vi "Test DAQ OPC and Robot.vi"(7 "error in":errorcluster) -> (0 "error out":errorcluster)   [LabVIEW 2013]
uses:
  SLL DAQ Engine/Software/Source Code/Sub VIs/DAQ Engine/Controls/SLL DE List of Digital Inputs.ctl
  SLL DAQ Engine/Software/Source Code/Sub VIs/DAQ Engine/Controls/SLL DE List of Digital Outputs.ctl
  Controls/ALTS-2015 Auto Program States.ctl
  Controls/ALTS-2015 Station Cluster.ctl
  Controls/ALTS-2015 Serial DB Details.ctl
  Controls/ALTS-2015 Serial Details.ctl
  Controls/ALTS-2015 Robot Tasks.ctl
  Controls/ALTS-2015 Robot FIFO Queue Options.ctl
  Controls/ALTS-2015 Task at Station Options.ctl
  Controls/ALTS-2015 LV2GBL Station Info Options.ctl
  SLL DAQ Engine/Software/Source Code/Sub VIs/DAQ Engine/Controls/SLL DE DI Global Options.ctl
  SLL DAQ Engine/Software/Source Code/Sub VIs/DAQ Engine/Controls/SLL DE DO Global Options.ctl
  Sub VIs/OPC Engine/Controls/ALTS-2015 OPC Write Global Options.ctl
  Sub VIs/OPC Engine/Controls/ALTS-2015 OPC Write Registers.ctl
  Sub VIs/OPC Engine/Controls/ALTS-2015 OPC Read Registers.ctl
  Sub VIs/OPC Engine/Controls/ALTS-2015 OPC Read Global Options.ctl
  Sub VIs/Robot Controller Queue/ALTS-2015 Robot Cotroller Options.ctl
  Globals/ALTS-2015 Global Variables.vi
panel:
  in  "Tab Control":T1(tab)
  out "History":string
  in  "STATION1 Start":bool
  in  "STATION1 Stop":bool
  in  "STATION1 Clamped":bool
  in  "STATION1 Test Type":T2(ring)=enum."Test Type 4"
  in  "STATION1 TC PASS":bool
  in  "STATION1 TC FAIL":bool
  in  "STATION1 Start DO":bool
  in  "Start Test":bool
  in  "Stop Test":bool
  in  "Scan Trigger":bool
  in  "Station No Start Stop Test":T3(ring)
  in  "Robot Available":bool
  out "Task Available for Robot?":bool
  out "New Serial Task?":bool
  out "Serial Adapter Plate Size":dbl
  out "Serial Displacement Size":dbl
  out "Serial Flange Size":dbl
  out "Test Result":bool
  out "Station Number":T3(ring)
  out "Rerun?":bool
  out "Invalid Serial Number":bool
  in  "PC ACK":bool
  in  "STATION3 Start":bool
  in  "STATION3 Stop":bool
  in  "STATION3 Clamped":bool
  in  "STATION3 Test Type":T2(ring)=enum."Test Type 4"
  in  "STATION3 TC PASS":bool
  in  "STATION3 TC FAIL":bool
  in  "STATION3 Start DO":bool
  in  "STATION2 Start":bool
  in  "STATION2 Stop":bool
  in  "STATION2 Clamped":bool
  in  "STATION2 Test Type":T2(ring)=enum."Test Type 4"
  in  "STATION2 TC PASS":bool
  in  "STATION2 TC FAIL":bool
  in  "STATION2 Start DO":bool
  in  "STATION4 Start":bool
  in  "STATION4 Stop":bool
  in  "STATION4 Clamped":bool
  in  "STATION4 Test Type":T2(ring)=enum."Test Type 4"
  in  "STATION4 TC PASS":bool
  in  "STATION4 TC FAIL":bool
  in  "STATION4 Start DO":bool
  in  "STATION1 Select Test":bool
  in  "STATION2 Select Test":bool
  in  "STATION3 Select Test":bool
  in  "STATION4 Select Test":bool
  out "Station No.":string[](array[string])=["Station 1", "Station 2", "Station 3", "Station 4"]
  out "Test Type":i32[](array[numeric])
  in  "STATION2 Stop DO":bool
  in  "STATION1 Stop DO":bool
  in  "STATION3 Stop DO":bool
  in  "STATION4 Stop DO":bool
  in  "STATION1 Light Indicator":enum16{"IDLE", "Test Running", "Pass", "Fail"}(ring)
  in  "STATION2 Light Indicator":enum16{"IDLE", "Test Running", "Pass", "Fail"}(ring)
  in  "STATION3 Light Indicator":enum16{"IDLE", "Test Running", "Pass", "Fail"}(ring)
  in  "STATION4 Light Indicator":enum16{"IDLE", "Test Running", "Pass", "Fail"}(ring)
  in  "Clear History":bool
  out "Serial Height":dbl
  out "Load Decision":dbl
  out "Cart Insert":dbl
  in  "Flush FIFO Queue":bool
  in  "Trigger Robot Controller State":bool
  in  "Roboto Controller State to Execute":T4=enum."Write Task Available for Robot"
  out "Load Serial Tasks":T5[](array[typedef])
  out "Invalid Serial Tasks":T5[](array[typedef])
  out "Rerun Serial Tasks":T5[](array[typedef])
  out "Unload Serial Tasks":T5[](array[typedef])
  out "# Unload Serial Tasks":i32
  out "# Rerun Serial Tasks":i32
  out "# Invalid Serial Tasks":i32
  out "# Load Serial Tasks":i32
  in  "New Serial Task Data":T9
  in  "Rerun Task Data":T10
  in  "Enqueue Invalid Serial":bool
  in  "Unload Task Data":T11
  out "All FIFO Elements":T5[](array[typedef])
  out "Current Station 1 Task":T5
  out "Current Station 2 Task":T5
  out "Current Station 3 Task":T5
  out "Current Station 4 Task":T5
  in  "Cart_Insert DS":dbl
  in  "Load_Decision DS":dbl
  in  "Serial_Height DS":dbl format="%.2g"
  in  "PC_ACK_Read_Tags DS":dbl
  out "DO Channel Name":T12
  in  "Invalid_SNo DS":dbl
  in  "Station_No_Start_Stop_Test DS":dbl
  in  "Start_Test DS":dbl
  in  "Rerun DS":dbl
  in  "Station_Number DS":dbl
  in  "Test_Result DS":dbl
  in  "Serial_Flange_Size DS":dbl
  in  "Serial_Displacement_Size DS":dbl
  in  "Serial_Adapter_Size DS":dbl
  in  "New_Serial DS":dbl
  in  "Scan_Trigger DS":dbl
  in  "Stop_Test DS":dbl
  in  "Task_Available_for_Robot DS":dbl
  in  "Robot_Available DS":dbl
  in  "DI Array":bool[](array[boolean])=[FALSE, FALSE, FALSE, FALSE, FALSE, FALSE, FALSE, FALSE, FALSE, FALSE, FALSE, FALSE, FALSE, FALSE, FALSE, FALSE, FALSE, FALSE, FALSE, FALSE, FALSE, FALSE, FALSE, FALSE, FALSE, FALSE, FALSE, FALSE]
  in  "DI Channel Name Array":T13[](array[typedef])=[enum."STATION1_START", enum."STATION1_STOP", enum."STATION1_CLAMPED", enum."STATION1_TC_PASS", enum."STATION1_TC_FAIL", enum."STATION1_TTA", enum."STATION1_TTB", enum."STATION2_START", enum."STATION2_STOP", enum."STATION2_CLAMPED", enum."STATION2_TC_PASS", enum."STATION2_TC_FAIL", enum."STATION2_TTA", enum."STATION2_TTB", enum."STATION3_START", enum."STATION3_STOP", enum."STATION3_CLAMPED", enum."STATION3_TC_PASS", enum."STATION3_TC_FAIL", enum."STATION3_TTA", enum."STATION3_TTB", enum."STATION4_START", enum."STATION4_STOP", enum."STATION4_CLAMPED", enum."STATION4_TC_PASS", enum."STATION4_TC_FAIL", enum."STATION4_TTA", enum."STATION4_TTB"]
  out "DO Channel Name Array":T12[](array[typedef])=[enum."STATION1_START TEST", enum."STATION1_STOP TEST", enum."STATION1_LIGHT1", enum."STATION1_LIGHT2", enum."STATION1_LIGHT3", enum."STATION1_SELECT_TEST", enum."STATION2_START TEST", enum."STATION2_STOP TEST", enum."STATION2_LIGHT1", enum."STATION2_LIGHT2", enum."STATION2_LIGHT3", enum."STATION2_SELECT_TEST", enum."STATION3_START TEST", enum."STATION3_STOP TEST", enum."STATION3_LIGHT1", enum."STATION3_LIGHT2", enum."STATION3_LIGHT3", enum."STATION3_SELECT_TEST", enum."STATION4_START TEST", enum."STATION4_STOP TEST", enum."STATION4_LIGHT1", enum."STATION4_LIGHT2", enum."STATION4_LIGHT3", enum."STATION4_SELECT_TEST"]
  out "DO Array":bool[](array[boolean])=[FALSE, FALSE, FALSE, FALSE, TRUE, FALSE, FALSE, FALSE, FALSE, FALSE, TRUE, FALSE, FALSE, FALSE, FALSE, FALSE, FALSE, FALSE, FALSE, FALSE, FALSE, FALSE, FALSE, FALSE]
  in  "DI Channel Name":T13
  # "ALTS-2015 Auto Mode Troubleshooter"
  # "Simulation VI to send DI Status and reads the DO output"
  # "Write Tags\nPC Writes to PLC\nPLC can only read these tags"
  # "Read Tags\nPC Reads from PLC"
  # "Test Type1: TTA:1, TTB: 0;\nTest Type2: TTA:0, TTB: 1;\nTest Type3: TTA:1, TTB: 1;\nTest Type4: TTA:0, TTB: 0;"
  # "IDLE : \t\t100\nTest Running:\t 010\nPass\t\t110\nFail\t\t101"
  # "STATION  1"
  # "STATION  2"
  # "Write Tags\nPC Writes to PLC\nPLC can only read these tags"
  # "Read Tags\nPC Reads from PLC"
  # "DI"
  # "DO"
  # "DI"
  # "DO"
  # "STATION  3"
  # "STATION  4"
  # "DI"
  # "DO"
  # "DI"
  # "DO"
  # "Invalid Serial Task Data"
  # "This tab indicates the tasks being executed at different station"
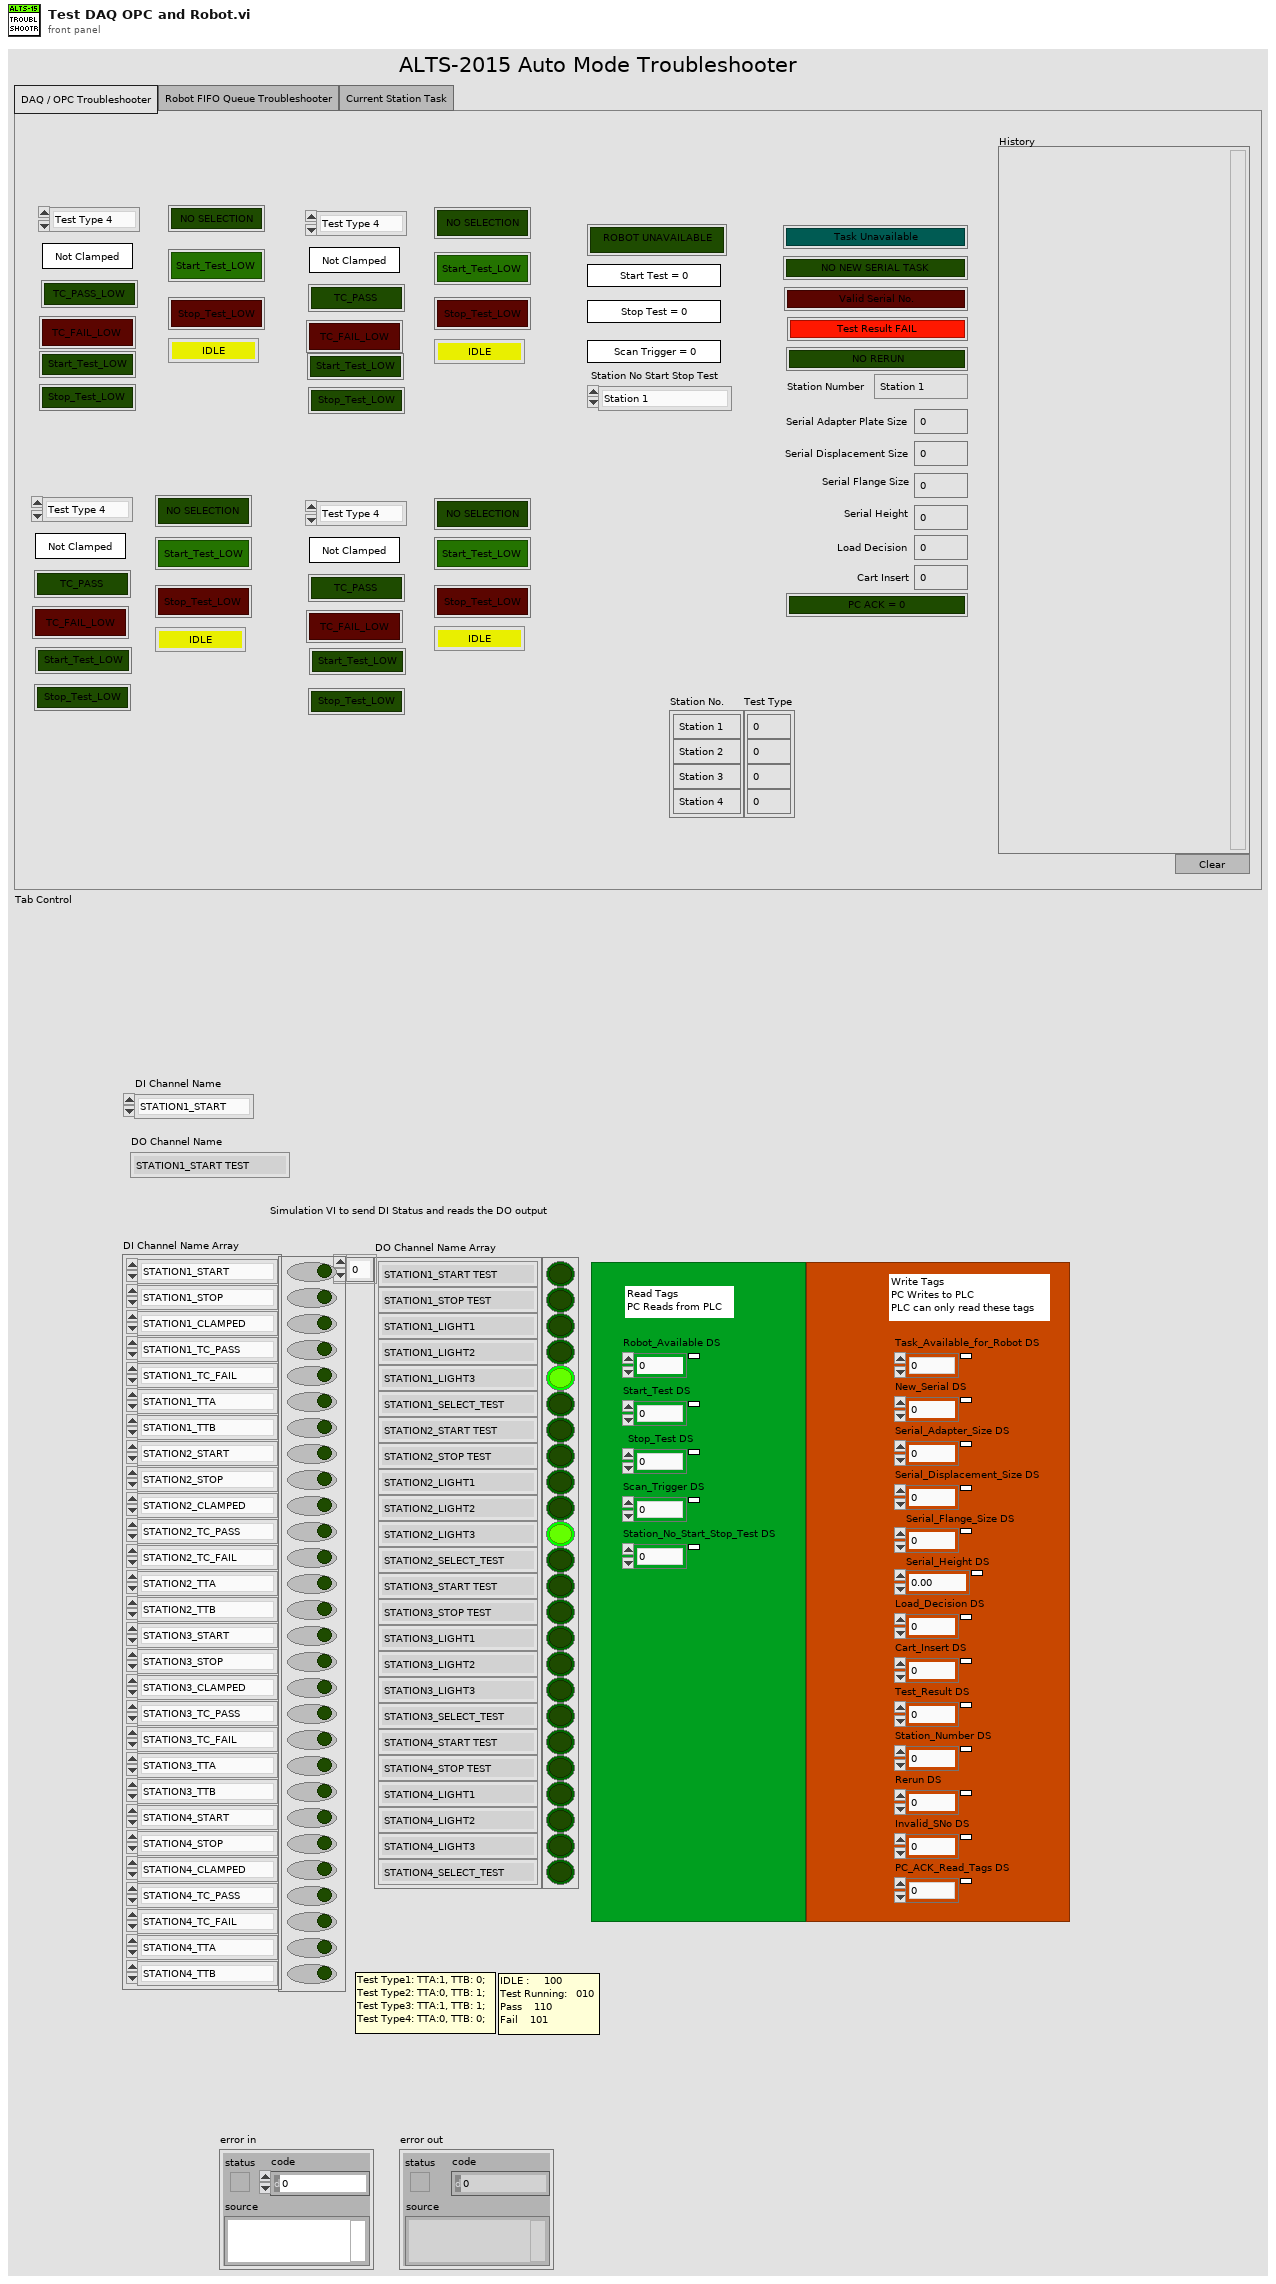
[diagram p1: front panel]
types:
  T1 = enum32{"DAQ / OPC Troubleshooter", "Robot FIFO Queue Troubleshooter", "Current Station Task"}
  T2 = enum16{"Test Type 1", "Test Type 2", "Test Type 3", "Test Type 4"}
  T3 = enum16{"Station 1", "Station 2", "Station 3", "Station 4"}
  T4 = typedef "ALTS-2015 Auto Program States.ctl" = enum16{"<------ Robot Handler States ------>", "Wait for Robot Availability", "Check Last Task by Robot", "Wait & Read Task from Queue", "Write New Task Details to Robot", "Write Task Available for Robot", "Check Robot for Unavailbilty", "Write Task Unavailable for Robot", "<------------ Other ------------>", "Error", "Exit"}
  T5 = typedef "ALTS-2015 Serial Details.ctl" = cluster{"Robot Task":T6, "Serial No":string, "New Serial?":bool, "Station # Unload":T7, "Last Test Result":bool, "Rerun?":bool, "Station # Rerun":T7, "Invalid Serial?":bool, "Serial Details":T8}
  T6 = typedef "ALTS-2015 Robot Tasks.ctl" = enum16{"Load", "Unload", "Rerun", "Invalid Serial"}
  T7 = typedef "ALTS-2015 Station Cluster.ctl" = enum16{"Station 1", "Station 2", "Station 3", "Station 4"}
  T8 = typedef "ALTS-2015 Serial DB Details.ctl" = cluster{"Adapter Plate Size":i32, "Air Leak Test Type ":i32, "Displacement Size":i32, "Flange Size":i32, "Height":i32, "Load Decision":i32, "Cart Insert":i32}
  T9 = cluster{"New Serial Details":T8, "Enqueue New Serial Task":bool}
  T10 = cluster{"Station # Rerun":T7, "Enqueue Rerun Task":bool}
  T11 = cluster{"Last Test Result":bool, "Station # Unload":T7, "Load Decision":i32, "Enqueue Unload Task":bool}
  T12 = typedef "SLL DE List of Digital Outputs.ctl" = enum16{"STATION1_START TEST", "STATION1_STOP TEST", "STATION1_LIGHT1", "STATION1_LIGHT2", "STATION1_LIGHT3", "STATION1_SELECT_TEST", "STATION2_START TEST", "STATION2_STOP TEST", "STATION2_LIGHT1", "STATION2_LIGHT2", "STATION2_LIGHT3", "STATION2_SELECT_TEST", "STATION3_START TEST", "STATION3_STOP TEST", "STATION3_LIGHT1", "STATION3_LIGHT2", "STATION3_LIGHT3", "STATION3_SELECT_TEST", "STATION4_START TEST", "STATION4_STOP TEST", "STATION4_LIGHT1", "STATION4_LIGHT2", "STATION4_LIGHT3", "STATION4_SELECT_TEST"}
  T13 = typedef "SLL DE List of Digital Inputs.ctl" = enum16{"STATION1_START", "STATION1_STOP", "STATION1_CLAMPED", "STATION1_TC_PASS", "STATION1_TC_FAIL", "STATION1_TTA", "STATION1_TTB", "STATION2_START", "STATION2_STOP", "STATION2_CLAMPED", "STATION2_TC_PASS", "STATION2_TC_FAIL", "STATION2_TTA", "STATION2_TTB", "STATION3_START", "STATION3_STOP", "STATION3_CLAMPED", "STATION3_TC_PASS", "STATION3_TC_FAIL", "STATION3_TTA", "STATION3_TTB", "STATION4_START", "STATION4_STOP", "STATION4_CLAMPED", "STATION4_TC_PASS", "STATION4_TC_FAIL", "STATION4_TTA", "STATION4_TTB"}
  T14 = enum32{"No PSP", "Read", "Write", "Write & Read"}
  T15 = typedef "ALTS-2015 INI Configuration Cluster.ctl" = cluster{"Application":cluster{"Rerun Count":i32, "Workorder No":string}, "Station Details":cluster{"Sensor Name 1":string, "Sensor Name 2":string, "Sensor Name 3":string, "Sensor Name 4":string, "Station1 Enable":bool, "Station2 Enable":bool, "Station3 Enable":bool, "Station4 Enable":bool}, "Database":cluster{"Database Connection Link":path, "Result Procedure":string, "User":string, "Password":string, "Prompt":bool, "Station 1 LT Result DB DSN Path":path, "Station 2 LT Result DB DSN Path":path, "Station 3 LT Result DB DSN Path":path, "Station 4 LT Result DB DSN Path":path, "AirLeakTestResult Procedure":string, "Serial Details Procedure":string}, "Simulation":cluster{"Simulate DAQ Hardware":bool, "Simulate Result DB Write":bool, "Simulate Scanner":bool, "Simulate OPC":bool, "Simulate Serial Details DB":bool, "Simulate Result DB":bool, "Simulate Scanner DB Path":path, "Simulate Serial Details DB Path":path, "Simulate Result DB Path":path}, "Barcode Scanner1":cluster{"Scanner IP":string, "Scanner Port":u16, "#Bytes to Read":i32}, "Barcode Scanner2":cluster{"Enabled?":bool, "Scanner IP":string, "Scanner Port":u16, "#Bytes to Read":i32}}
  T16 = typedef "SLL DE DO Global Options.ctl" = enum16{"Init", "Write Line", "Write Array", "Write Full Status", "Read Line", "Read Array", "Read Full Status", "Restart DO", "Send to Safe Mode", "Stop DO"}
  T17 = typedef "SLL DE DI Global Options.ctl" = enum16{"Init", "Write Line", "Write Array", "Read Line", "Read Array", "Read Full Status", "Write Full Status"}
  T18 = typedef "ALTS-2015 LV2GBL Station Info Options.ctl" = enum16{"Init", "Read", "Read All", "Write Sensor ID", "Write  Work Order", "Write Serial Number", "Write Test Data", "Write Station Status", "Write Station Occupancy", "Write Station Test Type", "Write Rerun", "Write Load Decision", "Write Robot Action", "Clear All", "Clear Test Result"}
  T19 = typedef "ALTS-2015 OPC Read Global Options.ctl" = enum16{"Init", "Write Value", "Write Array", "Read Value", "Read Array", "Read All"}
  T20 = typedef "ALTS-2015 OPC Write Global Options.ctl" = enum16{"Init", "Write Value", "Write Array", "Read Value", "Read Array", "Read All"}
  T21 = typedef "ALTS-2015 Robot Cotroller Options.ctl" = enum16{"Init", "Enqueue State", "Enqueue State in Opposite End", "Dequeue State", "Exit"}
  T22 = typedef "ALTS-2015 Robot FIFO Queue Options.ctl" = enum16{"Init", "Enqueue", "Dequeue", "Get Queue Elements", "Flush", "Destroy"}
  T23 = typedef "ALTS-2015 OPC Read Registers.ctl" = enum16{"Robot_Available", "Start_Test", "Stop_Test", "Scan_Trigger", "Station_No_Start_Stop_Test"}
  T24 = typedef "ALTS-2015 OPC Write Registers.ctl" = enum16{"Task_Available_for_Robot", "New_Serial", "Serial_Adapter_Size", "Serial_Displacement_Size", "Serial_Flange_Size", "Serial_Height", "Serial_LoadDecision", "Serial_CartInsert", "Test_Result", "Station_Number", "Rerun", "Invalid_SNo", "PC_ACK_Read_Tags"}
  T25 = typedef "ALTS-2015 Station Details.ctl" = cluster{"Station Number":string, "Work Order Number":string, "Sensor Name":string, "Pressure (PSI)":string, "Flow (SCCM)":string, "Test Time ":string, "Test Result":string, "Serial Number":string, "Station Status":T26, "SW assigned UUT":bool, "Rerun Count":i32, "Test Type":i32, "Load Decision":i32, "Robot Action":T27}
  T26 = typedef "ALTS-2015 Status Ring Indicator.ctl" = u16
  T27 = typedef "ALTS-2015 Robot Actions.ctl" = enum16{"Loading...", "Unloading...", "Reruning...", "No Action"}
  T28 = typedef "ALTS-2015 Task at Station Options.ctl" = enum16{"Init", "Write", "Read All", "Read"}
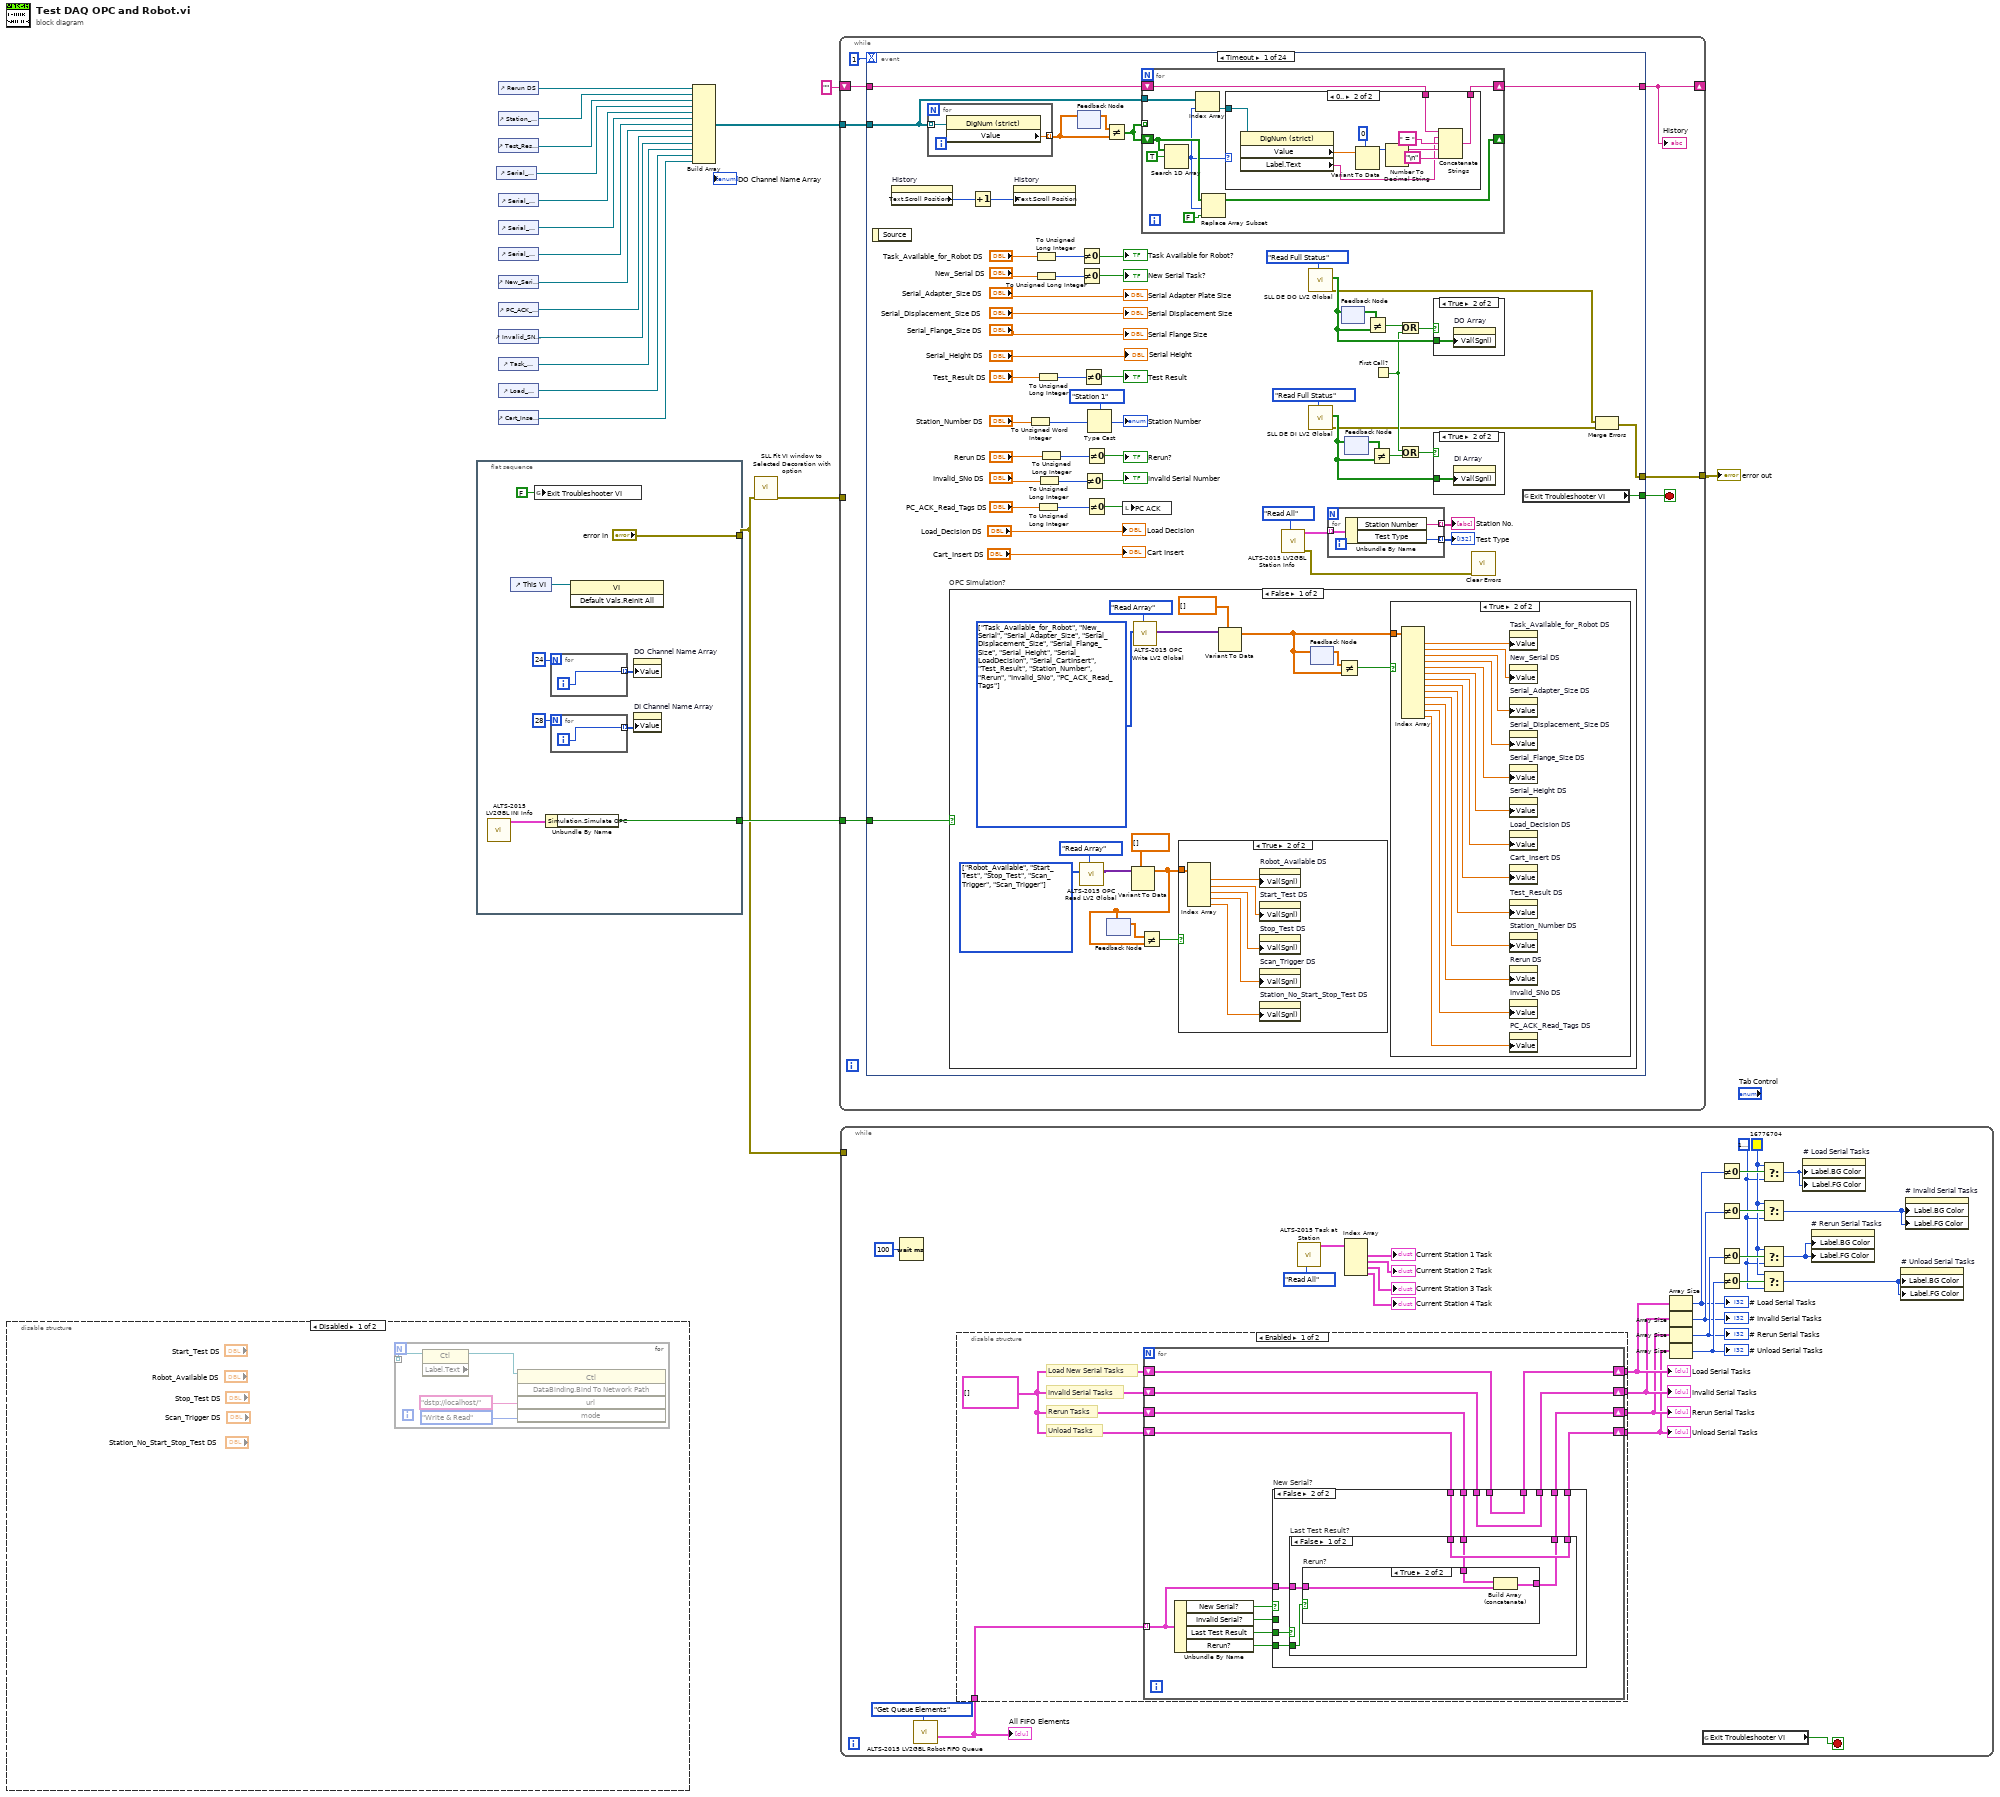
[diagram p0: block diagram]
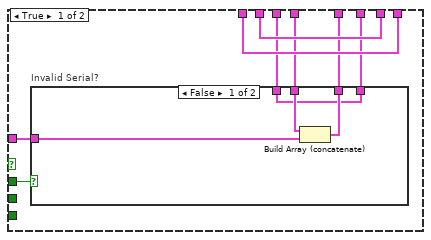
[diagram p2: hidden frame]
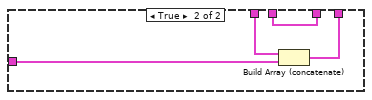
[diagram p3: hidden frame]
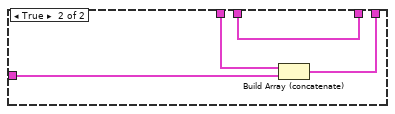
[diagram p5: hidden frame]
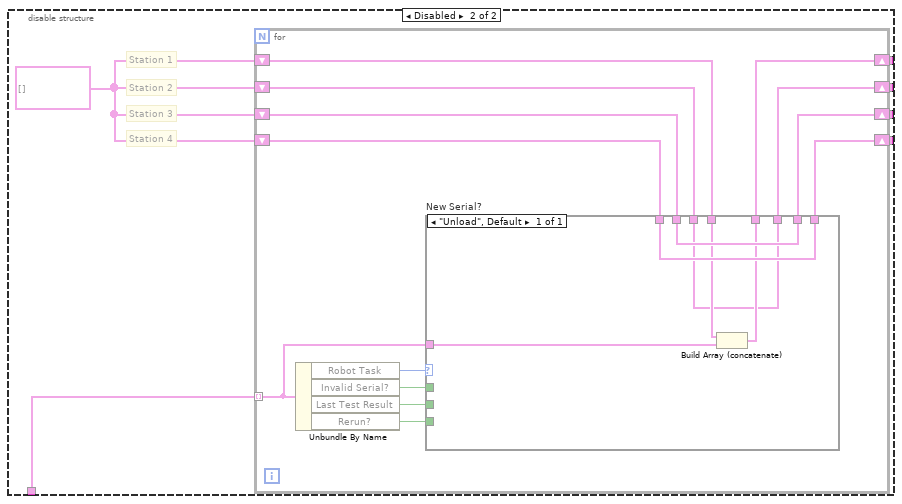
[diagram p6: hidden frame]
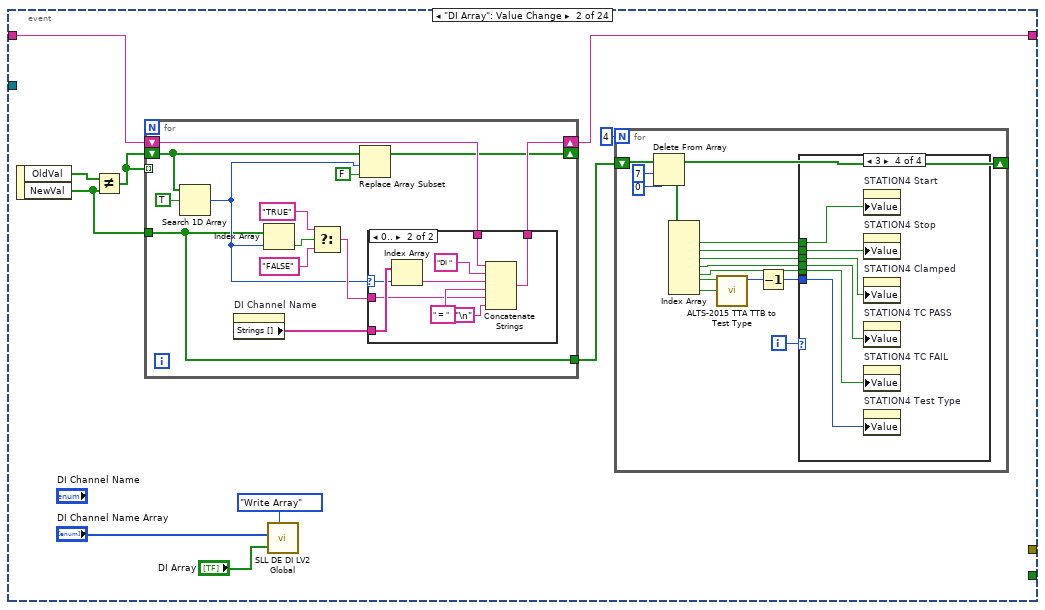
[diagram p13: hidden frame]
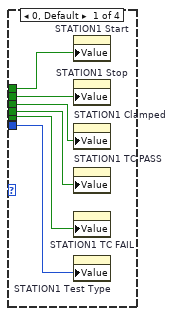
[diagram p14: hidden frame]
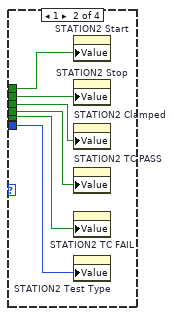
[diagram p15: hidden frame]
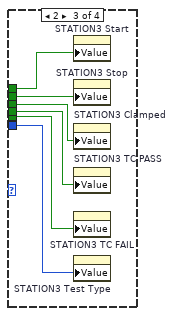
[diagram p16: hidden frame]
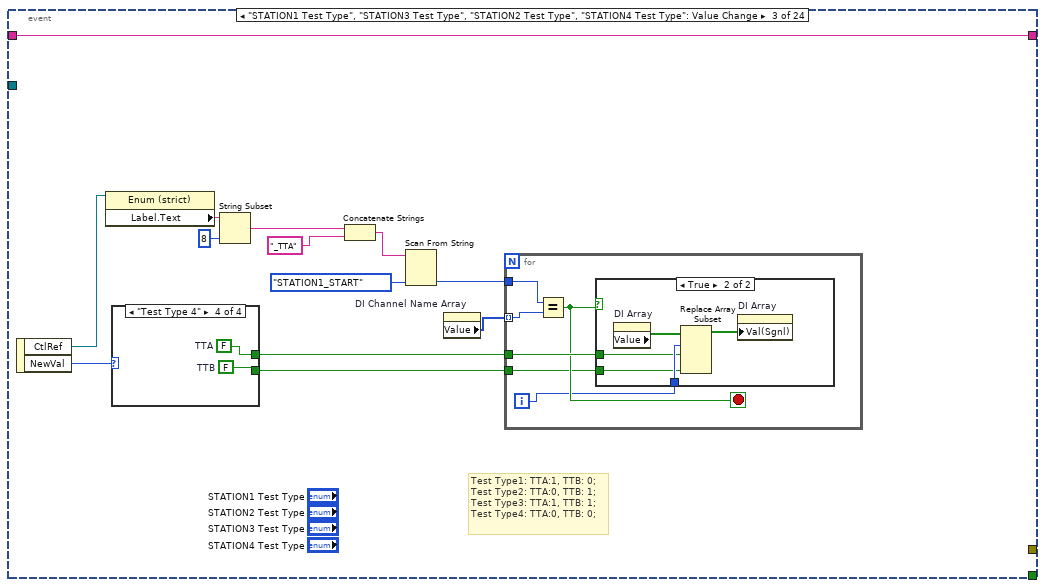
[diagram p18: hidden frame]
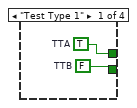
[diagram p19: hidden frame]
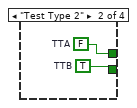
[diagram p20: hidden frame]
diagram:
  n1 = disable-structure shown="Disabled" {
    frame Disabled {
      n2 = for {
        tunnel: [w24] -> w20 mode=indexing
        n3 = property class="Ctl" props=["Label", "Text"](reference=w24) -> (reference out=w21:refnum<vi>)  [unwired: 1 in, 2 out]
        n4 = invoke on="Invoke Node" class="Ctl" method="DataBinding.Bind To Network Path"(reference=w21, "url"="dstp://localhost/" ("URL"), "mode"=T14."Write & Read" ("Mode")) -> ()  [unwired: 2 in, 5 out]
      }
    }
    frame Enabled {
    }
  }
  n5 = flat-sequence {
    tunnel: ["error in"] -> w1
    tunnel: [w25] -> w2
    frame #0 {
      n6 = call "ALTS-2015 LV2GBL INI Info.vi"() -> ("Configuration Cluster Out"=w26:T15)  [unwired: 10 in, 1 out]
      n7 = control-ref of="This VI"() -> (w31:refnum<vi>)
      n8 = global write "ALTS-2015 Global Variables.vi" "Exit Troubleshooter VI"(FALSE ("Exit Troubleshooter VI")) -> ()
      n9 = Unbundle By Name(w26) -> ("Simulation.Simulate OPC"=w25:bool)
      n10 = for {
        N: 24 -> [_]
        tunnel: [w35] -> w27 mode=indexing
        i -> [w35]
      }
      n11 = for {
        N: 28 -> [_]
        tunnel: [w34] -> w30 mode=indexing
        i -> [w34]
      }
      n12 = invoke class="VI" method="Default Vals.Reinit All"(reference=w31) -> ()  [unwired: 2 in, 3 out]
      n13 = property on="DO Channel Name Array" class="Arr (strict)"("Value"=w27) -> ()  [unwired: 2 in, 2 out]
      n14 = property on="DI Channel Name Array" class="Arr (strict)"("Value"=w30) -> ()  [unwired: 2 in, 2 out]
    }
  }
  n15 = control-ref of="Serial_Flange_Size DS"() -> (w17:refnum<vi>)
  n16 = control-ref of="Rerun DS"() -> (w14:refnum<vi>)
  n17 = control-ref of="Station_Number DS"() -> (w15:refnum<vi>)
  n18 = control-ref of="Test_Result DS"() -> (w16:refnum<vi>)
  n19 = control-ref of="Serial_Displacement_Size DS"() -> (w18:refnum<vi>)
  n20 = control-ref of="Serial_Adapter_Size DS"() -> (w19:refnum<vi>)
  n21 = control-ref of="Serial_Height DS"() -> (w9:refnum<vi>)
  n22 = control-ref of="New_Serial DS"() -> (w8:refnum<vi>)
  n23 = control-ref of="PC_ACK_Read_Tags DS"() -> (w7:refnum<vi>)
  n24 = control-ref of="Invalid_SNo DS"() -> (w6:refnum<vi>)
  n25 = control-ref of="Task_Available_for_Robot DS"() -> (w5:refnum<vi>)
  n26 = control-ref of="Load_Decision DS"() -> (w4:refnum<vi>)
  n27 = control-ref of="Cart_Insert DS"() -> (w3:refnum<vi>)
  n28 = Build Array(w14, w15, w16, w17, w18, w19, w9, w8, w7, w6, w5, w4, w3) -> (w11:refnum<vi>[])
  n29 = call "SLL Fit VI window to Selected Decoration with option.vi"("error in (no error)"=w1) -> ("error out"=w13:errorcluster)  [unwired: 9 in, 1 out]
  n30 = while {
    tunnel: w13 -> [_]
    tunnel: [w40] -> w10
    shift-right: [w38] -> _
    shift-left: "" -> [w39]
    tunnel: w11 -> [w37]
    tunnel: w2 -> [w36]
    stop <- w42 stop-if-true
    n31 = event shown="[0] Timeout" {
      selector: _ -> [_ _ _ _ _ _ _ _ _ _ _ _ _ _ _ _ _ _ _ _ _ _ _ _]
      dyn-events: _ -> [_ _ _ _ _ _ _ _ _ _ _ _ _ _ _ _ _ _ _ _ _ _ _ _]
      timeout: 1 -> [_ _ _ _ _ _ _ _ _ _ _ _ _ _ _ _ _ _ _ _ _ _ _ _]
      tunnel: [w77 _ _ _ _ _ _ _ _ _ _ _ _ _ _ _ _ _ _ _ _ _ _ _] -> w42
      tunnel: [w44 _ _ _ _ _ _ _ _ _ _ _ _ _ _ _ _ _ _ _ _ _ _ _] -> w40
      tunnel: [w65 w161 w233 w265 w285 w305 w325 w345 w366 w476 w511 w518 w521 w524 w527 w530 w534 w535 w538 w545 w553 w562 w570 ""] -> w38
      tunnel: w39 -> [w64 w162 w233 w265 w285 w305 w325 w345 w367 w476 w512 w518 w521 w524 w527 w530 w534 w535 w538 w545 w553 w562 w570 _]
      tunnel: w37 -> [w63 _ _ _ _ _ _ _ _ _ _ _ _ _ _ _ _ _ _ _ _ _ _ _]
      tunnel: w36 -> [w49 _ _ _ _ _ _ _ _ _ _ _ _ _ _ _ _ _ _ _ _ _ _ _]
      event Timeout {
        n32 = event-data() -> ()  [unwired: 1 in, 1 out]
        n33 = property on="History" class="Str"() -> ("Text.Scroll Position"=w62:u32)  [unwired: 2 in, 2 out]
        n34 = for {
          tunnel: w63 -> [w156] mode=indexing
          tunnel: [w155] -> w53 mode=indexing
          n35 = property class="DigNum (strict)"(reference=w156) -> ("Value"=w155:dbl)  [unwired: 1 in, 2 out]
        }
        n36 = case "OPC Simulation?" shown="False" w49 {
          frame False {
            w109 = T23[] [enum."Robot_Available", enum."Start_Test", enum."Stop_Test", enum."Scan_Trigger", enum."Scan_Trigger"] items=["Robot_Available", "Start_Test", "Stop_Test", "Scan_Trigger", "Station_No_Start_Stop_Test"] ("OPC Read Register Array")
            w110 = T24[] [enum."Task_Available_for_Robot", enum."New_Serial", enum."Serial_Adapter_Size", enum."Serial_Displacement_Size", enum."Serial_Flange_Size", enum."Serial_Height", enum."Serial_LoadDecision", enum."Serial_CartInsert", enum."Test_Result", enum."Station_Number", enum."Rerun", enum."Invalid_SNo", enum."PC_ACK_Read_Tags"] items=["Task_Available_for_Robot", "New_Serial", "Serial_Adapter_Size", "Serial_Displacement_Size", "Serial_Flange_Size", "Serial_Height", "Serial_LoadDecision", "Serial_CartInsert", "Test_Result", "Station_Number", "Rerun", "Invalid_SNo", "PC_ACK_Read_Tags"] ("OPC Write Register Array")
            n37 = call "ALTS-2015 OPC Read LV2 Global.vi"("Options"=ALTS-2015_OPC_Read_Global_Options."Read Array", "OPC Read Register Array"=w109) -> ("OPC Read Register Array Value"=w106:variant[])  [unwired: 7 in, 2 out]
            n38 = feedback #1() -> (w105:dbl[])  [unwired: 1 in]
            n39 = Variant To Data(type=dbl[] [], Variant=w106) -> (data=w103:dbl[])  [unwired: 1 in, 1 out]
            n40 = feedback-in #1(w103) -> ()
            n41 = call "ALTS-2015 OPC Write LV2 Global.vi"("Options"=ALTS-2015_OPC_Write_Global_Options."Read Array", "OPC Write Register Array"=w110) -> ("OPC Read Register Array Value"=w112:variant[])  [unwired: 7 in, 2 out]
            n42 = Not Equal?(x=w105, y=w103) -> (x != y?=w101:bool)
            n43 = case shown="True" w101 {
              tunnel: w103 -> [_ w128]
              frame False {
              }
              frame True {
                n44 = Index Array(array=w128) -> (element #1=w133:dbl, element #2=w132:dbl, element #3=w131:dbl, element #4=w130:dbl, element #5=w129:dbl)  [unwired: 5 in]
                n45 = property on="Robot_Available DS" class="DigNum (strict)"("Val(Sgnl)"=w133) -> ()  [unwired: 2 in, 2 out]
                n46 = property on="Start_Test DS" class="DigNum (strict)"("Val(Sgnl)"=w132) -> ()  [unwired: 2 in, 2 out]
                n47 = property on="Stop_Test DS" class="DigNum (strict)"("Val(Sgnl)"=w131) -> ()  [unwired: 2 in, 2 out]
                n48 = property on="Scan_Trigger DS" class="DigNum (strict)"("Val(Sgnl)"=w130) -> ()  [unwired: 2 in, 2 out]
                n49 = property on="Station_No_Start_Stop_Test DS" class="DigNum (strict)"("Val(Sgnl)"=w129) -> ()  [unwired: 2 in, 2 out]
              }
            }
            n50 = Variant To Data(type=dbl[] [], Variant=w112) -> (data=w102:dbl[])  [unwired: 1 in, 1 out]
            n51 = feedback #2() -> (w104:dbl[])  [unwired: 1 in]
            n52 = feedback-in #2(w102) -> ()
            n53 = Not Equal?(x=w104, y=w102) -> (x != y?=w100:bool)
            n54 = case shown="True" w100 {
              tunnel: w102 -> [_ w114]
              frame False {
              }
              frame True {
                n55 = Index Array(array=w114) -> (element #1=w115:dbl, element #2=w116:dbl, element #3=w117:dbl, element #4=w118:dbl, element #5=w119:dbl, element #6=w120:dbl, element #7=w121:dbl, element #8=w122:dbl, element #9=w123:dbl, element #10=w124:dbl, element #11=w125:dbl, element #12=w126:dbl, element #13=w127:dbl)  [unwired: 13 in]
                n56 = property on="Task_Available_for_Robot DS" class="DigNum (strict)"("Value"=w115) -> ()  [unwired: 2 in, 2 out]
                n57 = property on="New_Serial DS" class="DigNum (strict)"("Value"=w116) -> ()  [unwired: 2 in, 2 out]
                n58 = property on="Serial_Adapter_Size DS" class="DigNum (strict)"("Value"=w117) -> ()  [unwired: 2 in, 2 out]
                n59 = property on="Serial_Displacement_Size DS" class="DigNum (strict)"("Value"=w118) -> ()  [unwired: 2 in, 2 out]
                n60 = property on="Serial_Flange_Size DS" class="DigNum (strict)"("Value"=w119) -> ()  [unwired: 2 in, 2 out]
                n61 = property on="Serial_Height DS" class="DigNum (strict)"("Value"=w120) -> ()  [unwired: 2 in, 2 out]
                n62 = property on="Load_Decision DS" class="DigNum (strict)"("Value"=w121) -> ()  [unwired: 2 in, 2 out]
                n63 = property on="Cart_Insert DS" class="DigNum (strict)"("Value"=w122) -> ()  [unwired: 2 in, 2 out]
                n64 = property on="Test_Result DS" class="DigNum (strict)"("Value"=w123) -> ()  [unwired: 2 in, 2 out]
                n65 = property on="Station_Number DS" class="DigNum (strict)"("Value"=w124) -> ()  [unwired: 2 in, 2 out]
                n66 = property on="Rerun DS" class="DigNum (strict)"("Value"=w125) -> ()  [unwired: 2 in, 2 out]
                n67 = property on="Invalid_SNo DS" class="DigNum (strict)"("Value"=w126) -> ()  [unwired: 2 in, 2 out]
                n68 = property on="PC_ACK_Read_Tags DS" class="DigNum (strict)"("Value"=w127) -> ()  [unwired: 2 in, 2 out]
              }
            }
          }
          frame True {
          }
        }
        n69 = Increment(x=w62) -> (x+1=w61:u32)
        n70 = property on="History" class="Str"("Text.Scroll Position"=w61) -> ()  [unwired: 2 in, 2 out]
        n71 = To Unsigned Word Integer(number="Station_Number DS") -> (unsigned 16bit integer=w80:u16)
        n72 = To Unsigned Long Integer(number="Task_Available_for_Robot DS") -> (unsigned 32bit integer=w97:u32)
        n73 = To Unsigned Long Integer(number="New_Serial DS") -> (unsigned 32bit integer=w96:u32)
        n74 = To Unsigned Long Integer(number="Test_Result DS") -> (unsigned 32bit integer=w90:u32)
        n75 = To Unsigned Long Integer(number="PC_ACK_Read_Tags DS") -> (unsigned 32bit integer=w58:u32)
        n76 = To Unsigned Long Integer(number="Invalid_SNo DS") -> (unsigned 32bit integer=w83:u32)
        n77 = To Unsigned Long Integer(number="Rerun DS") -> (unsigned 32bit integer=w86:u32)
        n78 = feedback-in #3(w53) -> ()
        n79 = feedback #3() -> (w52:dbl[])  [unwired: 1 in]
        n80 = Not Equal To 0?(x=w97) -> (x != 0?=→"Task Available for Robot?":bool)
        n81 = Not Equal To 0?(x=w96) -> (x != 0?=→"New Serial Task?":bool)
        n82 = Not Equal To 0?(x=w90) -> (x != 0?=→"Test Result":bool)
        n83 = Not Equal To 0?(x=w83) -> (x != 0?=→"Invalid Serial Number":bool)
        n84 = Not Equal To 0?(x=w86) -> (x != 0?=→"Rerun?":bool)
        n85 = Not Equal To 0?(x=w58) -> (x != 0?=w60:bool)
        n86 = Type Cast(type=T3."Station 1" ("Station Number"), x=w80) -> (*(type *) &x=→"Station Number":T3)
        n87 = Not Equal?(x=w52, y=w53) -> (x != y?=w66:bool[])
        n88 = local write "PC ACK"(w60) -> ()
        n89 = for {
          shift-right: [w138] -> _
          shift-left: w66 -> [w139]
          tunnel: w66 -> [_] mode=indexing
          shift-right: [w141] -> w65
          shift-left: w64 -> [w142]
          tunnel: w63 -> [w135]
          n90 = Search 1D Array(1D array=w139, element=TRUE) -> (index of element=w137:i32)  [unwired: 1 in]
          n91 = Index Array(array=w135, index=w137) -> (element=w140:refnum<vi>)
          n92 = Replace Array Subset(array=w139, new element=FALSE ("new element/subarray"), index=w137) -> (w138:bool[])
          n93 = case shown="0.." w137 {
            tunnel: [w144 w153] -> w141
            tunnel: w142 -> [w144 w152]
            tunnel: w140 -> [_ w147]
            frame -1, Default {
            }
            frame 0.. {
              n94 = property class="DigNum (strict)"(reference=w147) -> ("Value"=w151:dbl, "Label.Text"=w148:string)  [unwired: 1 in, 2 out]
              n95 = Variant To Data(type=0 ("concatenated string"), Variant=w151) -> (data=w145:i32)  [unwired: 1 in, 1 out]
              n96 = Number To Decimal String(number=w145) -> (decimal integer string=w150:string)  [unwired: 1 in]
              n97 = Concatenate Strings(w152, w148, " = " ("string"), w150, "\n") -> (w153:string)
            }
          }
        }
        n98 = call "ALTS-2015 LV2GBL Station Info.vi"("Options"=ALTS-2015_LV2GBL_Station_Info_Options."Read All") -> ("error out"=w72:errorcluster, "Station Info Array"=w74:T25[])  [unwired: 8 in, 1 out]
        n99 = call "SLL DE DO LV2 Global.vi"("DO Option"=SLL_DE_DO_Global_Options."Read Full Status") -> ("error out"=w43:errorcluster, "Digital Array Status"=w55:bool[])  [unwired: 7 in, 2 out]
        n100 = call "SLL DE DI LV2 Global.vi"("Option"=SLL_DE_DI_Global_Options."Read Full Status") -> ("error out"=w45:errorcluster, "Digital Array Status"=w70:bool[])  [unwired: 7 in, 2 out]
        n101 = for {
          tunnel: w74 -> [w160] mode=indexing
          tunnel: [w159] -> w76 mode=indexing
          tunnel: [w158] -> w75 mode=indexing
          n102 = Unbundle By Name(w160) -> ("Station Number"=w158:string, "Test Type"=w159:i32)
        }
        "Station No." <- w75
        "Test Type" <- w76
        n103 = feedback #4() -> (w56:bool[])  [unwired: 1 in]
        n104 = feedback-in #4(w55) -> ()
        n105 = feedback #5() -> (w68:bool[])  [unwired: 1 in]
        n106 = feedback-in #5(w70) -> ()
        n107 = Not Equal?(x=w56, y=w55) -> (x != y?=w57:bool)
        n108 = Not Equal?(x=w68, y=w70) -> (x != y?=w69:bool)
        n109 = First Call?() -> (First Call?: T/F=w46:bool)
        n110 = Or(x=w57, y=w46) -> (x .or. y?=w48:bool)
        n111 = Or(x=w46, y=w69) -> (x .or. y?=w47:bool)
        n112 = case shown="True" w48 {
          tunnel: w55 -> [_ w134]
          frame False {
          }
          frame True {
            n113 = property on="DO Array" class="Arr (strict)"("Val(Sgnl)"=w134) -> ()  [unwired: 2 in, 2 out]
          }
        }
        n114 = case shown="True" w47 {
          tunnel: w70 -> [_ w157]
          frame False {
          }
          frame True {
            n115 = property on="DI Array" class="Arr (strict)"("Val(Sgnl)"=w157) -> ()  [unwired: 2 in, 2 out]
          }
        }
        n116 = call <vilib>:"Clear Errors.vi"("error in (no error)"=w72) -> ()  [unwired: 6 in, 1 out]
        n117 = global read "ALTS-2015 Global Variables.vi" "Exit Troubleshooter VI"() -> (w77:bool)
        n118 = Merge Errors(w43, w45) -> (w44:errorcluster)
        "Serial Adapter Plate Size" <- "Serial_Adapter_Size DS"
        "Serial Displacement Size" <- "Serial_Displacement_Size DS"
        "Serial Flange Size" <- "Serial_Flange_Size DS"
        "Serial Height" <- "Serial_Height DS"
        "Cart Insert" <- "Cart_Insert DS"
        "Load Decision" <- "Load_Decision DS"
      }
      event "DI Array": Value Change {
        n119 = event-data() -> ("OldVal"=w164:bool[], "NewVal"=w163:bool[])  [unwired: 1 in]
        n120 = Not Equal?(x=w164, y=w163) -> (x != y?=w165:bool[])
        n121 = for {
          shift-right: [w215] -> _
          shift-left: w165 -> [w216]
          shift-right: [w221] -> w161
          shift-left: w162 -> [w220]
          tunnel: w165 -> [_] mode=indexing
          tunnel: w163 -> [w210]
          tunnel: [w210] -> w167
          n122 = Search 1D Array(1D array=w216, element=TRUE) -> (index of element=w212:i32)  [unwired: 1 in]
          n123 = property on="DI Channel Name" class="Enum (strict)"() -> ("Strings []"=w211:string[])  [unwired: 2 in, 2 out]
          n124 = Index Array(array=w210, index=w212) -> (element=w219:bool)
          n125 = Select(t="TRUE", s=w219, f="FALSE") -> (s? t:f=w213:string)
          n126 = Replace Array Subset(array=w216, new element=FALSE ("new element/subarray"), index=w212) -> (w215:bool[])
          n127 = case shown="0.." w212 {
            selector: w212 -> [_ w224]
            tunnel: w211 -> [_ w232]
            tunnel: [w223 w230] -> w221
            tunnel: w220 -> [w223 w229]
            tunnel: w213 -> [_ w227]
            frame -1, Default {
            }
            frame 0.. {
              n128 = Index Array(array=w232, index=w224) -> (element=w231:string)
              n129 = Concatenate Strings(w229, "DI " ("string"), w231, " = " ("string"), w227, "\n") -> (w230:string)
            }
          }
        }
        n130 = call "SLL DE DI LV2 Global.vi"("DI State Array"="DI Array", "Option"=SLL_DE_DI_Global_Options."Write Array", "DI Channel Name Array"="DI Channel Name Array") -> ()  [unwired: 5 in, 4 out]
        n131 = for {
          N: 4 -> [_]
          shift-right: [w181] -> _
          shift-left: w167 -> [w185]
          i -> [w172]
          n132 = Delete From Array(array=w185, length=7, index=0) -> (deleted portion=w182:bool[], array with subset deleted=w181:bool[])
          n133 = Index Array(array=w182) -> (element #1=w177:bool, element #2=w176:bool, element #3=w174:bool, element #4=w173:bool, element #5=w175:bool, element #6=w180:bool, element #7=w179:bool)  [unwired: 7 in]
          n134 = call "ALTS-2015 TTA TTB to Test Type.vi"("TTB"=w179, "TTA"=w180) -> ("Test Type"=w178:i32)  [unwired: 9 in]
          n135 = Decrement(x=w178) -> (x-1=w171:i32)
          n136 = case shown="3" w172 {
            tunnel: w171 -> [w191 w197 w203 w209]
            tunnel: w177 -> [w190 w196 w202 w208]
            tunnel: w176 -> [w189 w195 w201 w207]
            tunnel: w175 -> [w188 w194 w200 w206]
            tunnel: w174 -> [w187 w193 w199 w205]
            tunnel: w173 -> [w186 w192 w198 w204]
            frame 0, Default {
              n137 = property on="STATION1 Start" class="Bool (strict)"("Value"=w190) -> ()  [unwired: 2 in, 2 out]
              n138 = property on="STATION1 Stop" class="Bool (strict)"("Value"=w189) -> ()  [unwired: 2 in, 2 out]
              n139 = property on="STATION1 Clamped" class="Bool (strict)"("Value"=w187) -> ()  [unwired: 2 in, 2 out]
              n140 = property on="STATION1 TC PASS" class="Bool (strict)"("Value"=w186) -> ()  [unwired: 2 in, 2 out]
              n141 = property on="STATION1 TC FAIL" class="Bool (strict)"("Value"=w188) -> ()  [unwired: 2 in, 2 out]
              n142 = property on="STATION1 Test Type" class="Enum (strict)"("Value"=w191) -> ()  [unwired: 2 in, 2 out]
            }
            frame 1 {
              n143 = property on="STATION2 Start" class="Bool (strict)"("Value"=w196) -> ()  [unwired: 2 in, 2 out]
              n144 = property on="STATION2 Stop" class="Bool (strict)"("Value"=w195) -> ()  [unwired: 2 in, 2 out]
              n145 = property on="STATION2 Clamped" class="Bool (strict)"("Value"=w193) -> ()  [unwired: 2 in, 2 out]
              n146 = property on="STATION2 TC PASS" class="Bool (strict)"("Value"=w192) -> ()  [unwired: 2 in, 2 out]
              n147 = property on="STATION2 TC FAIL" class="Bool (strict)"("Value"=w194) -> ()  [unwired: 2 in, 2 out]
              n148 = property on="STATION2 Test Type" class="Enum (strict)"("Value"=w197) -> ()  [unwired: 2 in, 2 out]
            }
            frame 2 {
              n149 = property on="STATION3 Start" class="Bool (strict)"("Value"=w202) -> ()  [unwired: 2 in, 2 out]
              n150 = property on="STATION3 Stop" class="Bool (strict)"("Value"=w201) -> ()  [unwired: 2 in, 2 out]
              n151 = property on="STATION3 Clamped" class="Bool (strict)"("Value"=w199) -> ()  [unwired: 2 in, 2 out]
              n152 = property on="STATION3 TC PASS" class="Bool (strict)"("Value"=w198) -> ()  [unwired: 2 in, 2 out]
              n153 = property on="STATION3 TC FAIL" class="Bool (strict)"("Value"=w200) -> ()  [unwired: 2 in, 2 out]
              n154 = property on="STATION3 Test Type" class="Enum (strict)"("Value"=w203) -> ()  [unwired: 2 in, 2 out]
            }
            frame 3 {
              n155 = property on="STATION4 Start" class="Bool (strict)"("Value"=w208) -> ()  [unwired: 2 in, 2 out]
              n156 = property on="STATION4 Stop" class="Bool (strict)"("Value"=w207) -> ()  [unwired: 2 in, 2 out]
              n157 = property on="STATION4 Clamped" class="Bool (strict)"("Value"=w205) -> ()  [unwired: 2 in, 2 out]
              n158 = property on="STATION4 TC PASS" class="Bool (strict)"("Value"=w204) -> ()  [unwired: 2 in, 2 out]
              n159 = property on="STATION4 TC FAIL" class="Bool (strict)"("Value"=w206) -> ()  [unwired: 2 in, 2 out]
              n160 = property on="STATION4 Test Type" class="Enum (strict)"("Value"=w209) -> ()  [unwired: 2 in, 2 out]
            }
          }
        }
      }
      event "STATION1 Test Type", "STATION3 Test Type", "STATION2 Test Type", "STATION4 Test Type": Value Change {
        # "Test Type1: TTA:1, TTB: 0;\nTest Type2: TTA:0, TTB: 1;\nTest Type3: TTA:1, TTB: 1;\nTest Type4: TTA:0, TTB: 0;"
        n161 = event-data() -> ("CtlRef"=w238:refnum<vi>, "NewVal"=w243:T2)  [unwired: 1 in]
        n162 = property class="Enum (strict)"(reference=w238) -> ("Label.Text"=w240:string)  [unwired: 1 in, 2 out]
        n163 = case shown="\"Test Type 4\"" w243 {
          tunnel: [w247 w249 w251 w253] -> w242
          tunnel: [w246 w248 w250 w252] -> w241
          frame "Test Type 1" {
            w246 = FALSE  # TTB
            w247 = TRUE  # TTA
          }
          frame "Test Type 2" {
            w248 = TRUE  # TTB
            w249 = FALSE  # TTA
          }
          frame "Test Type 3" {
            w250 = TRUE  # TTB
            w251 = TRUE  # TTA
          }
          frame "Test Type 4" {
            w252 = FALSE  # TTB
            w253 = FALSE  # TTA
          }
        }
        n164 = String Subset(string=w240, length (rest)=8 ("length (rest)")) -> (substring=w239:string)  [unwired: 1 in]
        n165 = Concatenate Strings(w239, "_TTA" ("string")) -> (w236:string)
        n166 = Scan From String(input string=w236, default 1=SLL_DE_List_of_Digital_Inputs."STATION1_START" ("List of Digital Inputs")) -> (output 1=w235:T13)  [unwired: 3 in, 3 out]
        n167 = property on="DI Channel Name Array" class="Arr (strict)"() -> ("Value"=w244:T13[])  [unwired: 2 in, 2 out]
        n168 = for {
          tunnel: w235 -> [w259]
          tunnel: w244 -> [w258] mode=indexing
          tunnel: w242 -> [w257]
          tunnel: w241 -> [w254]
          i -> [w255]
          stop <- w256 stop-if-true
          n169 = Equal?(x=w259, y=w258) -> (x = y?=w256:bool)
          n170 = case shown="True" w256 {
            tunnel: w255 -> [_ w263]
            tunnel: w257 -> [_ w261]
            tunnel: w254 -> [_ w260]
            frame False {
            }
            frame True {
              n171 = property on="DI Array" class="Arr (strict)"() -> ("Value"=w264:bool[])  [unwired: 2 in, 2 out]
              n172 = Replace Array Subset(array=w264, new element #1=w261, index #1=w263, new element #2=w260) -> (w262:bool[])  [unwired: 1 in]
              n173 = property on="DI Array" class="Arr (strict)"("Val(Sgnl)"=w262) -> ()  [unwired: 2 in, 2 out]
            }
          }
        }
      }
      event "STATION1 Clamped", "STATION3 Clamped", "STATION2 Clamped", "STATION4 Clamped": Value Change {
        n174 = event-data() -> ("CtlRef"=w272:refnum<vi>, "NewVal"=w273:bool)  [unwired: 1 in]
        n175 = property class="Bool (strict)"(reference=w272) -> ("Label.Text"=w271:string)  [unwired: 1 in, 2 out]
        n176 = String Subset(string=w271, length (rest)=8 ("length (rest)")) -> (substring=w270:string)  [unwired: 1 in]
        n177 = Concatenate Strings(w270, "_CLAMPED" ("string")) -> (w268:string)
        n178 = property on="DI Channel Name Array" class="Arr (strict)"() -> ("Value"=w274:T13[])  [unwired: 2 in, 2 out]
        n179 = Scan From String(input string=w268, default 1=SLL_DE_List_of_Digital_Inputs."STATION1_START" ("List of Digital Inputs")) -> (output 1=w267:T13)  [unwired: 3 in, 3 out]
        n180 = for {
          tunnel: w267 -> [w280]
          tunnel: w274 -> [w279] mode=indexing
          tunnel: w273 -> [w276]
          i -> [w278]
          stop <- w277 stop-if-true
          n181 = Equal?(x=w280, y=w279) -> (x = y?=w277:bool)
          n182 = case shown="True" w277 {
            tunnel: w278 -> [_ w283]
            tunnel: w276 -> [_ w281]
            frame False {
            }
            frame True {
              n183 = property on="DI Array" class="Arr (strict)"() -> ("Value"=w284:bool[])  [unwired: 2 in, 2 out]
              n184 = Replace Array Subset(array=w284, new element=w281, index=w283) -> (w282:bool[])
              n185 = property on="DI Array" class="Arr (strict)"("Val(Sgnl)"=w282) -> ()  [unwired: 2 in, 2 out]
            }
          }
        }
      }
      event "STATION1 TC PASS", "STATION3 TC PASS", "STATION2 TC PASS", "STATION4 TC PASS": Value Change {
        n186 = event-data() -> ("CtlRef"=w289:refnum<vi>, "NewVal"=w293:bool)  [unwired: 1 in]
        n187 = property class="Bool (strict)"(reference=w289) -> ("Label.Text"=w291:string)  [unwired: 1 in, 2 out]
        n188 = String Subset(string=w291, length (rest)=8 ("length (rest)")) -> (substring=w290:string)  [unwired: 1 in]
        n189 = Concatenate Strings(w290, "_TC_PASS" ("string")) -> (w288:string)
        n190 = property on="DI Channel Name Array" class="Arr (strict)"() -> ("Value"=w294:T13[])  [unwired: 2 in, 2 out]
        n191 = Scan From String(input string=w288, default 1=SLL_DE_List_of_Digital_Inputs."STATION1_START" ("List of Digital Inputs")) -> (output 1=w286:T13)  [unwired: 3 in, 3 out]
        n192 = for {
          tunnel: w286 -> [w300]
          tunnel: w294 -> [w299] mode=indexing
          tunnel: w293 -> [w296]
          i -> [w298]
          stop <- w297 stop-if-true
          n193 = Equal?(x=w300, y=w299) -> (x = y?=w297:bool)
          n194 = case shown="True" w297 {
            tunnel: w298 -> [_ w303]
            tunnel: w296 -> [_ w301]
            frame False {
            }
            frame True {
              n195 = property on="DI Array" class="Arr (strict)"() -> ("Value"=w304:bool[])  [unwired: 2 in, 2 out]
              n196 = Replace Array Subset(array=w304, new element=w301, index=w303) -> (w302:bool[])
              n197 = property on="DI Array" class="Arr (strict)"("Val(Sgnl)"=w302) -> ()  [unwired: 2 in, 2 out]
            }
          }
        }
      }
      event "STATION1 TC FAIL", "STATION3 TC FAIL", "STATION2 TC FAIL", "STATION4 TC FAIL": Value Change {
        n198 = event-data() -> ("CtlRef"=w310:refnum<vi>, "NewVal"=w313:bool)  [unwired: 1 in]
        n199 = property class="Bool (strict)"(reference=w310) -> ("Label.Text"=w311:string)  [unwired: 1 in, 2 out]
        n200 = String Subset(string=w311, length (rest)=8 ("length (rest)")) -> (substring=w309:string)  [unwired: 1 in]
        n201 = property on="DI Channel Name Array" class="Arr (strict)"() -> ("Value"=w314:T13[])  [unwired: 2 in, 2 out]
        n202 = Concatenate Strings(w309, "_TC_FAIL" ("string")) -> (w308:string)
        n203 = Scan From String(input string=w308, default 1=SLL_DE_List_of_Digital_Inputs."STATION1_START" ("List of Digital Inputs")) -> (output 1=w306:T13)  [unwired: 3 in, 3 out]
        n204 = for {
          tunnel: w314 -> [w320] mode=indexing
          tunnel: w313 -> [w317]
          tunnel: w306 -> [w316]
          i -> [w319]
          stop <- w318 stop-if-true
          n205 = Equal?(x=w316, y=w320) -> (x = y?=w318:bool)
          n206 = case shown="True" w318 {
            tunnel: w319 -> [_ w323]
            tunnel: w317 -> [_ w321]
            frame False {
            }
            frame True {
              n207 = property on="DI Array" class="Arr (strict)"() -> ("Value"=w324:bool[])  [unwired: 2 in, 2 out]
              n208 = Replace Array Subset(array=w324, new element=w321, index=w323) -> (w322:bool[])
              n209 = property on="DI Array" class="Arr (strict)"("Val(Sgnl)"=w322) -> ()  [unwired: 2 in, 2 out]
            }
          }
        }
      }
      event "STATION1 Start", "STATION2 Start", "STATION3 Start", "STATION4 Start": Value Change {
        n210 = event-data() -> ("CtlRef"=w332:refnum<vi>, "NewVal"=w333:bool)  [unwired: 1 in]
        n211 = property class="Bool (strict)"(reference=w332) -> ("Label.Text"=w331:string)  [unwired: 1 in, 2 out]
        n212 = String Subset(string=w331, length (rest)=8 ("length (rest)")) -> (substring=w329:string)  [unwired: 1 in]
        n213 = property on="DI Channel Name Array" class="Arr (strict)"() -> ("Value"=w334:T13[])  [unwired: 2 in, 2 out]
        n214 = Concatenate Strings(w329, "_START" ("string")) -> (w328:string)
        n215 = Scan From String(input string=w328, default 1=SLL_DE_List_of_Digital_Inputs."STATION1_START" ("List of Digital Inputs")) -> (output 1=w326:T13)  [unwired: 3 in, 3 out]
        n216 = for {
          tunnel: w326 -> [w340]
          tunnel: w334 -> [w339] mode=indexing
          tunnel: w333 -> [w336]
          i -> [w338]
          stop <- w337 stop-if-true
          n217 = Equal?(x=w340, y=w339) -> (x = y?=w337:bool)
          n218 = case shown="True" w337 {
            tunnel: w338 -> [_ w343]
            tunnel: w336 -> [_ w341]
            frame False {
            }
            frame True {
              n219 = property on="DI Array" class="Arr (strict)"() -> ("Value"=w344:bool[])  [unwired: 2 in, 2 out]
              n220 = Replace Array Subset(array=w344, new element=w341, index=w343) -> (w342:bool[])
              n221 = property on="DI Array" class="Arr (strict)"("Val(Sgnl)"=w342) -> ()  [unwired: 2 in, 2 out]
            }
          }
        }
      }
      event "STATION1 Stop", "STATION2 Stop", "STATION3 Stop", "STATION4 Stop": Value Change {
        n222 = event-data() -> ("CtlRef"=w352:refnum<vi>, "NewVal"=w353:bool)  [unwired: 1 in]
        n223 = property class="Bool (strict)"(reference=w352) -> ("Label.Text"=w351:string)  [unwired: 1 in, 2 out]
        n224 = String Subset(string=w351, length (rest)=8 ("length (rest)")) -> (substring=w350:string)  [unwired: 1 in]
        n225 = property on="DI Channel Name Array" class="Arr (strict)"() -> ("Value"=w354:T13[])  [unwired: 2 in, 2 out]
        n226 = Concatenate Strings(w350, "_STOP" ("string")) -> (w348:string)
        n227 = Scan From String(input string=w348, default 1=SLL_DE_List_of_Digital_Inputs."STATION1_START" ("List of Digital Inputs")) -> (output 1=w347:T13)  [unwired: 3 in, 3 out]
        n228 = for {
          tunnel: w347 -> [w360]
          tunnel: w354 -> [w359] mode=indexing
          tunnel: w353 -> [w356]
          i -> [w358]
          stop <- w357 stop-if-true
          n229 = Equal?(x=w360, y=w359) -> (x = y?=w357:bool)
          n230 = case shown="True" w357 {
            tunnel: w358 -> [_ w363]
            tunnel: w356 -> [_ w361]
            frame False {
            }
            frame True {
              n231 = property on="DI Array" class="Arr (strict)"() -> ("Value"=w364:bool[])  [unwired: 2 in, 2 out]
              n232 = Replace Array Subset(array=w364, new element=w361, index=w363) -> (w362:bool[])
              n233 = property on="DI Array" class="Arr (strict)"("Val(Sgnl)"=w362) -> ()  [unwired: 2 in, 2 out]
            }
          }
        }
      }
      event "DO Array": Value Change {
        n234 = event-data() -> ("NewVal"=w365:bool[], "OldVal"=w370:bool[])  [unwired: 1 in]
        n235 = property on="DO Channel Name Array" class="Arr (strict)"() -> ("Value"=w369:T12[])  [unwired: 2 in, 2 out]
        n236 = Not Equal?(x=w365, y=w370) -> (x != y?=w368:bool[])
        n237 = for {
          tunnel: w368 -> [w396] mode=indexing
          tunnel: w369 -> [w395] mode=indexing
          tunnel: w365 -> [w394]
          n238 = case shown="True" w396 {
            tunnel: w395 -> [_ w402]
            tunnel: w394 -> [_ w397]
            frame False {
            }
            frame True {
              # "IDLE : \t\t100\nTest Running:\t 010\nPass\t\t110\nFail\t\t101"
              n239 = Format Into String(format string="%s", w402) -> (resulting string=w398:string)  [unwired: 2 in, 1 out]
              n240 = String Subset(string=w398, offset (0)=9 ("length (rest)")) -> (substring=w399:string)  [unwired: 1 in]
              n241 = case shown="\"START TEST\", Default" w399 {
                tunnel: w397 -> [w411 w420 w429 w459]
                frame "START TEST", Default {
                  n242 = Index Array(array=w411, index #1=0 ("index"), index #2=6 ("index"), index #3=12 ("index"), index #4=18 ("index")) -> (element #1=w406:bool, element #2=w405:bool, element #3=w404:bool, element #4=w403:bool)
                  n243 = property on="STATION1 Start DO" class="Bool (strict)"("Value"=w406) -> ()  [unwired: 2 in, 2 out]
                  n244 = property on="STATION2 Start DO" class="Bool (strict)"("Value"=w405) -> ()  [unwired: 2 in, 2 out]
                  n245 = property on="STATION3 Start DO" class="Bool (strict)"("Value"=w404) -> ()  [unwired: 2 in, 2 out]
                  n246 = property on="STATION4 Start DO" class="Bool (strict)"("Value"=w403) -> ()  [unwired: 2 in, 2 out]
                }
                frame "STOP TEST" {
                  n247 = Index Array(array=w420, index #1=1 ("index"), index #2=7 ("index"), index #3=13 ("index"), index #4=19 ("index")) -> (element #1=w415:bool, element #2=w414:bool, element #3=w413:bool, element #4=w412:bool)
                  n248 = property on="STATION1 Stop DO" class="Bool (strict)"("Value"=w415) -> ()  [unwired: 2 in, 2 out]
                  n249 = property on="STATION2 Stop DO" class="Bool (strict)"("Value"=w414) -> ()  [unwired: 2 in, 2 out]
                  n250 = property on="STATION3 Stop DO" class="Bool (strict)"("Value"=w413) -> ()  [unwired: 2 in, 2 out]
                  n251 = property on="STATION4 Stop DO" class="Bool (strict)"("Value"=w412) -> ()  [unwired: 2 in, 2 out]
                }
                frame "SELECT_TEST" {
                  n252 = Index Array(array=w429, index #1=5 ("index"), index #2=11 ("index"), index #3=17 ("index"), index #4=23 ("index")) -> (element #1=w424:bool, element #2=w423:bool, element #3=w422:bool, element #4=w421:bool)
                  n253 = property on="STATION1 Select Test" class="Bool (strict)"("Value"=w424) -> ()  [unwired: 2 in, 2 out]
                  n254 = property on="STATION2 Select Test" class="Bool (strict)"("Value"=w423) -> ()  [unwired: 2 in, 2 out]
                  n255 = property on="STATION3 Select Test" class="Bool (strict)"("Value"=w422) -> ()  [unwired: 2 in, 2 out]
                  n256 = property on="STATION4 Select Test" class="Bool (strict)"("Value"=w421) -> ()  [unwired: 2 in, 2 out]
                }
                frame "LIGHT1", "LIGHT2", "LIGHT3" {
                  w442 = "%d%d%d" ("format string")
                  n257 = Index Array(array=w459, index #1=2 ("index"), index #4=8 ("index"), index #7=14 ("index"), index #10=20 ("index")) -> (element #1=w454:bool, element #2=w453:bool, element #3=w452:bool, element #4=w451:bool, element #5=w450:bool, element #6=w449:bool, element #7=w448:bool, element #8=w447:bool, element #9=w445:bool, element #10=w446:bool, element #11=w444:bool, element #12=w443:bool)  [unwired: 8 in]
                  n258 = Format Into String(format string=w442, w454, w453, w452) -> (resulting string=w441:string)  [unwired: 2 in, 1 out]
                  n259 = Format Into String(format string=w442, w451, w450, w449) -> (resulting string=w438:string)  [unwired: 2 in, 1 out]
                  n260 = Format Into String(format string=w442, w448, w447, w445) -> (resulting string=w436:string)  [unwired: 2 in, 1 out]
                  n261 = Format Into String(format string=w442, w446, w444, w443) -> (resulting string=w434:string)  [unwired: 2 in, 1 out]
                  n262 = Reverse String(1:w441) -> (0:w440:string)
                  n263 = Reverse String(1:w438) -> (0:w439:string)
                  n264 = Reverse String(1:w436) -> (0:w437:string)
                  n265 = Reverse String(1:w434) -> (0:w435:string)
                  n266 = case shown="\"110\"" w440 {
                    tunnel: [enum16{"IDLE", "Test Running", "Pass", "Fail"}."IDLE" ("STATION1 Light Indicator") enum16{"IDLE", "Test Running", "Pass", "Fail"}."Test Running" ("STATION1 Light Indicator") enum16{"IDLE", "Test Running", "Pass", "Fail"}."Pass" ("STATION1 Light Indicator") enum16{"IDLE", "Test Running", "Pass", "Fail"}."Fail" ("STATION1 Light Indicator")] -> w433
                    frame "100", Default {
                    }
                    frame "010" {
                    }
                    frame "110" {
                    }
                    frame "101" {
                    }
                  }
                  n267 = case shown="\"110\"" w439 {
                    tunnel: [enum16{"IDLE", "Test Running", "Pass", "Fail"}."IDLE" ("STATION1 Light Indicator") enum16{"IDLE", "Test Running", "Pass", "Fail"}."Test Running" ("STATION1 Light Indicator") enum16{"IDLE", "Test Running", "Pass", "Fail"}."Pass" ("STATION1 Light Indicator") enum16{"IDLE", "Test Running", "Pass", "Fail"}."Fail" ("STATION1 Light Indicator")] -> w432
                    frame "100", Default {
                    }
                    frame "010" {
                    }
                    frame "110" {
                    }
                    frame "101" {
                    }
                  }
                  n268 = case shown="\"110\"" w437 {
                    tunnel: [enum16{"IDLE", "Test Running", "Pass", "Fail"}."IDLE" ("STATION1 Light Indicator") enum16{"IDLE", "Test Running", "Pass", "Fail"}."Test Running" ("STATION1 Light Indicator") enum16{"IDLE", "Test Running", "Pass", "Fail"}."Pass" ("STATION1 Light Indicator") enum16{"IDLE", "Test Running", "Pass", "Fail"}."Fail" ("STATION1 Light Indicator")] -> w431
                    frame "100", Default {
                    }
                    frame "010" {
                    }
                    frame "110" {
                    }
                    frame "101" {
                    }
                  }
                  n269 = case shown="\"110\"" w435 {
                    tunnel: [enum16{"IDLE", "Test Running", "Pass", "Fail"}."IDLE" ("STATION1 Light Indicator") enum16{"IDLE", "Test Running", "Pass", "Fail"}."Test Running" ("STATION1 Light Indicator") enum16{"IDLE", "Test Running", "Pass", "Fail"}."Pass" ("STATION1 Light Indicator") enum16{"IDLE", "Test Running", "Pass", "Fail"}."Fail" ("STATION1 Light Indicator")] -> w430
                    frame "100", Default {
                    }
                    frame "010" {
                    }
                    frame "110" {
                    }
                    frame "101" {
                    }
                  }
                  n270 = property on="STATION1 Light Indicator" class="Enum (strict)"("Value"=w433) -> ()  [unwired: 2 in, 2 out]
                  n271 = property on="STATION2 Light Indicator" class="Enum (strict)"("Value"=w432) -> ()  [unwired: 2 in, 2 out]
                  n272 = property on="STATION3 Light Indicator" class="Enum (strict)"("Value"=w431) -> ()  [unwired: 2 in, 2 out]
                  n273 = property on="STATION4 Light Indicator" class="Enum (strict)"("Value"=w430) -> ()  [unwired: 2 in, 2 out]
                }
              }
            }
          }
        }
        n274 = for {
          shift-right: [w375] -> _
          shift-left: w368 -> [w374]
          shift-right: [w372] -> w366
          shift-left: w367 -> [w373]
          tunnel: w368 -> [_] mode=indexing
          tunnel: w365 -> [w371]
          n275 = Search 1D Array(1D array=w374, element=TRUE) -> (index of element=w381:i32)  [unwired: 1 in]
          n276 = property on="DO Channel Name" class="Enum (strict)"() -> ("Strings []"=w383:string[])  [unwired: 2 in, 2 out]
          n277 = Index Array(array=w371, index=w381) -> (element=w377:bool)
          n278 = Select(t="TRUE", s=w377, f="FALSE") -> (s? t:f=w380:string)
          n279 = Replace Array Subset(array=w374, new element=FALSE ("new element/subarray"), index=w381) -> (w375:bool[])
          n280 = case shown="0.." w381 {
            selector: w381 -> [_ w385]
            tunnel: [w384 w392] -> w372
            tunnel: w383 -> [_ w391]
            tunnel: w373 -> [w384 w390]
            tunnel: w380 -> [_ w388]
            frame -1, Default {
            }
            frame 0.. {
              n281 = Index Array(array=w391, index=w385) -> (element=w393:string)
              n282 = Concatenate Strings(w390, "DO " ("string"), w393, " = " ("string"), w388, "\n") -> (w392:string)
            }
          }
        }
      }
      event "STATION1 Select Test", "STATION2 Select Test", "STATION3 Select Test", "STATION4 Select Test", "STATION1 Light Indicator", "STATION2 Light Indicator", "STATION3 Light Indicator", "STATION4 Light Indicator", "STATION1 Start DO", "STATION2 Start DO", "STATION3 Start DO", "STATION4 Start DO", "STATION1 Stop DO", "STATION2 Stop DO", "STATION3 Stop DO", "STATION4 Stop DO": Value Change {
        n283 = event-data() -> ()  [unwired: 1 in, 6 out]
        n284 = for {
          N: 4 -> [_]
          shift-right: [w489] -> w478
          shift-left: bool[] [] -> [w482]
          i -> [w483]
          # "IDLE : \t\t100\nTest Running:\t 010\nPass\t\t110\nFail\t\t101"
          n285 = case shown="0, Default" w483 {
            tunnel: ["STATION1 Start DO" "STATION2 Start DO" "STATION3 Start DO" "STATION4 Start DO"] -> w488
            tunnel: ["STATION1 Stop DO" "STATION2 Stop DO" "STATION3 Stop DO" "STATION4 Stop DO"] -> w487
            tunnel: ["STATION1 Select Test" "STATION2 Select Test" "STATION3 Select Test" "STATION4 Select Test"] -> w485
            tunnel: ["STATION1 Light Indicator" "STATION2 Light Indicator" "STATION3 Light Indicator" "STATION4 Light Indicator"] -> w484
            frame 0, Default {
            }
            frame 1 {
            }
            frame 2 {
            }
            frame 3 {
            }
          }
          n286 = case shown="\"Fail\"" w484 {
            tunnel: [bool[] [FALSE, FALSE, TRUE] ("DO State Array") bool[] [FALSE, TRUE, FALSE] ("DO State Array") bool[] [FALSE, TRUE, TRUE] ("DO State Array") bool[] [TRUE, FALSE, TRUE] ("DO State Array")] -> w486
            frame "IDLE", Default {
            }
            frame "Test Running" {
            }
            frame "Pass" {
            }
            frame "Fail" {
            }
          }
          n287 = Build Array (concatenate)(w482, w488, w487, w486, w485) -> (w489:bool[])
        }
        n288 = property on="DO Channel Name Array" class="Arr (strict)"() -> ("Value"=w480:T12[])  [unwired: 2 in, 2 out]
        n289 = call "SLL DE DO LV2 Global.vi"("DO State Array"=w478, "DO Option"=SLL_DE_DO_Global_Options."Write Array", "DO Channel Name Array"=w480) -> ()  [unwired: 5 in, 4 out]
      }
      event "Robot_Available DS", "Start_Test DS", "Stop_Test DS", "Scan_Trigger DS", "Station_No_Start_Stop_Test DS": Value Change {
        n290 = event-data() -> ("CtlRef"=w510:refnum<vi>)  [unwired: 1 in, 5 out]
        n291 = property class="DigNum (strict)"(reference=w510) -> ("Label.Text"=w513:string, "Value"=w514:dbl)  [unwired: 1 in, 2 out]
        n292 = Number To Decimal String(number=w514) -> (decimal integer string=w515:string)  [unwired: 1 in]
        n293 = Concatenate Strings(w512, w513, " = " ("string"), w515, "\n") -> (w511:string)
      }
      event "Robot Available": Value Change {
        n294 = event-data() -> ()  [unwired: 1 in, 6 out]
        n295 = Boolean To (0,1)(Boolean="Robot Available") -> (0, 1=w519:i16)
        n296 = property on="Robot_Available DS" class="DigNum (strict)"("Val(Sgnl)"=w519) -> ()  [unwired: 2 in, 2 out]
      }
      event "Start Test": Value Change {
        n297 = event-data() -> ("NewVal"=w523:bool)  [unwired: 1 in, 5 out]
        n298 = Boolean To (0,1)(Boolean=w523) -> (0, 1=w522:i16)
        n299 = property on="Start_Test DS" class="DigNum (strict)"("Val(Sgnl)"=w522) -> ()  [unwired: 2 in, 2 out]
      }
      event "Stop Test": Value Change {
        n300 = event-data() -> ("NewVal"=w526:bool)  [unwired: 1 in, 5 out]
        n301 = Boolean To (0,1)(Boolean=w526) -> (0, 1=w525:i16)
        n302 = property on="Stop_Test DS" class="DigNum (strict)"("Val(Sgnl)"=w525) -> ()  [unwired: 2 in, 2 out]
      }
      event "Scan Trigger": Value Change {
        n303 = event-data() -> ("NewVal"=w529:bool)  [unwired: 1 in]
        n304 = Boolean To (0,1)(Boolean=w529) -> (0, 1=w528:i16)
        n305 = property on="Scan_Trigger DS" class="DigNum (strict)"("Val(Sgnl)"=w528) -> ()  [unwired: 2 in, 2 out]
      }
      event "Station No Start Stop Test": Value Change {
        n306 = event-data() -> ("NewVal"=w531:T3)  [unwired: 1 in]
        n307 = property on="Station_No_Start_Stop_Test DS" class="DigNum (strict)"("Val(Sgnl)"=w531) -> ()  [unwired: 2 in, 2 out]
      }
      event "PC ACK": Value Change {
        n308 = event-data() -> ()  [unwired: 1 in, 6 out]
        n309 = Boolean To (0,1)(Boolean="PC ACK") -> (0, 1=w532:i16)
        n310 = property on="PC_ACK_Read_Tags DS" class="DigNum (strict)"("Val(Sgnl)"=w532) -> ()  [unwired: 2 in, 2 out]
      }
      event "Trigger Robot Controller State": Value Change {
        n311 = event-data() -> ()  [unwired: 1 in, 6 out]
        n312 = call "ALTS-2015 Robot State Controller.vi"("Option"=ALTS-2015_Robot_Cotroller_Options."Enqueue State", "Enqueue State"="Roboto Controller State to Execute") -> ()  [unwired: 8 in, 2 out]
      }
      event "Enqueue Invalid Serial": Value Change {
        w541 = T5 {"Robot Task"=enum."Load", "Serial No"="", "New Serial?"=FALSE, "Station # Unload"=enum."Station 1", "Last Test Result"=FALSE, "Rerun?"=FALSE, "Station # Rerun"=enum."Station 1", "Invalid Serial?"=FALSE, "Serial Details"={"Adapter Plate Size"=0, "Air Leak Test Type "=0, "Displacement Size"=0, "Flange Size"=0, "Height"=0, "Load Decision"=0, "Cart Insert"=0}}  # Task Details
        n313 = event-data() -> ()  [unwired: 1 in, 6 out]
        n314 = Bundle By Name(cluster=w541, "New Serial?"=TRUE ("New Part?"), "Invalid Serial?"=TRUE) -> (w539:T5)
        n315 = call "ALTS-2015 LV2GBL Robot FIFO Queue.vi"("Options"=ALTS-2015_Robot_FIFO_Queue_Options."Enqueue" ("Enum"), "Task Details In"=w539) -> ()  [unwired: 5 in, 5 out]
      }
      event "Unload Task Data.Enqueue Unload Task": Value Change {
        w546 = T5 {"Robot Task"=enum."Load", "Serial No"="", "New Serial?"=FALSE, "Station # Unload"=enum."Station 1", "Last Test Result"=FALSE, "Rerun?"=FALSE, "Station # Rerun"=enum."Station 1", "Invalid Serial?"=FALSE, "Serial Details"={"Adapter Plate Size"=0, "Air Leak Test Type "=0, "Displacement Size"=0, "Flange Size"=0, "Height"=0, "Load Decision"=0, "Cart Insert"=0}}  # Task Details
        n316 = event-data() -> ()  [unwired: 1 in, 6 out]
        n317 = Unbundle By Name("Unload Task Data") -> ("Station # Unload"=w551:T7, "Last Test Result"=w552:bool, "Load Decision"=w544:i32)
        n318 = Bundle By Name(cluster=w546, "New Serial?"=FALSE ("New Part?"), "Station # Unload"=w551, "Last Test Result"=w552, "Serial Details.Load Decision"=w544) -> (w549:T5)
        n319 = call "ALTS-2015 LV2GBL Robot FIFO Queue.vi"("Options"=ALTS-2015_Robot_FIFO_Queue_Options."Enqueue" ("Enum"), "Task Details In"=w549) -> ()  [unwired: 5 in, 5 out]
      }
      event "Rerun Task Data.Enqueue Rerun Task": Value Change {
        w554 = T5 {"Robot Task"=enum."Load", "Serial No"="", "New Serial?"=FALSE, "Station # Unload"=enum."Station 1", "Last Test Result"=FALSE, "Rerun?"=FALSE, "Station # Rerun"=enum."Station 1", "Invalid Serial?"=FALSE, "Serial Details"={"Adapter Plate Size"=0, "Air Leak Test Type "=0, "Displacement Size"=0, "Flange Size"=0, "Height"=0, "Load Decision"=0, "Cart Insert"=0}}  # Task Details
        n320 = event-data() -> ()  [unwired: 1 in, 6 out]
        n321 = Unbundle By Name("Rerun Task Data") -> ("Station # Rerun"=w561:T7)
        n322 = Bundle By Name(cluster=w554, "New Serial?"=FALSE ("New Part?"), "Rerun?"=TRUE, "Station # Rerun"=w561, "Last Test Result"=FALSE) -> (w557:T5)
        n323 = call "ALTS-2015 LV2GBL Robot FIFO Queue.vi"("Options"=ALTS-2015_Robot_FIFO_Queue_Options."Enqueue" ("Enum"), "Task Details In"=w557) -> ()  [unwired: 5 in, 5 out]
      }
      event "New Serial Task Data.Enqueue New Serial Task": Value Change {
        w565 = T5 {"Robot Task"=enum."Load", "Serial No"="", "New Serial?"=FALSE, "Station # Unload"=enum."Station 1", "Last Test Result"=FALSE, "Rerun?"=FALSE, "Station # Rerun"=enum."Station 1", "Invalid Serial?"=FALSE, "Serial Details"={"Adapter Plate Size"=0, "Air Leak Test Type "=0, "Displacement Size"=0, "Flange Size"=0, "Height"=0, "Load Decision"=0, "Cart Insert"=0}}  # Task Details
        n324 = event-data() -> ()  [unwired: 1 in, 6 out]
        n325 = Unbundle By Name("New Serial Task Data") -> ("New Serial Details"=w563:T8)
        n326 = Bundle By Name(cluster=w565, "New Serial?"=TRUE ("New Part?"), "Serial Details"=w563) -> (w568:T5)
        n327 = call "ALTS-2015 LV2GBL Robot FIFO Queue.vi"("Options"=ALTS-2015_Robot_FIFO_Queue_Options."Enqueue" ("Enum"), "Task Details In"=w568) -> ()  [unwired: 5 in, 5 out]
      }
      event "Flush FIFO Queue": Value Change {
        n328 = event-data() -> ()  [unwired: 1 in, 6 out]
        n329 = call "ALTS-2015 LV2GBL Robot FIFO Queue.vi"("Options"=ALTS-2015_Robot_FIFO_Queue_Options."Flush" ("Enum")) -> ()  [unwired: 6 in, 5 out]
      }
      event "Clear History": Value Change {
        n330 = event-data() -> ()  [unwired: 1 in, 6 out]
      }
    }
    "History" <- w38
  }
  "error out" <- w10
  n331 = while {
    tunnel: w1 -> [_]
    stop <- w593 stop-if-true
    w583 = u32 16776704
    w582 = u32 16777216
    n332 = Wait (ms)(milliseconds to wait=u32 100) -> ()  [unwired: 1 out]
    n333 = call "ALTS-2015 LV2GBL Robot FIFO Queue.vi"("Options"=ALTS-2015_Robot_FIFO_Queue_Options."Get Queue Elements" ("Enum")) -> ("elements"=w598:T5[])  [unwired: 6 in, 4 out]
    "All FIFO Elements" <- w598
    n334 = disable-structure shown="Enabled" {
      disable-tunnel: w598 -> [w605 w662]
      disable-tunnel: [w604 w661] -> w597
      disable-tunnel: [w603 w660] -> w596
      disable-tunnel: [w602 w659] -> w595
      disable-tunnel: [w601 w658] -> w594
      frame Enabled {
        w600 = T5[] []
        # "Unload Tasks"
        # "Rerun Tasks"
        # "Invalid Serial Tasks"
        # "Load New Serial Tasks"
        n335 = for {
          tunnel: w605 -> [w616] mode=indexing
          shift-right: [w617] -> w604
          shift-left: w600 -> [w618]
          shift-right: [w613] -> w603
          shift-left: w600 -> [w612]
          shift-right: [w606] -> w602
          shift-left: w600 -> [w607]
          shift-right: [w610] -> w601
          shift-left: w600 -> [w611]
          n336 = Unbundle By Name(w616) -> ("New Serial?"=w615:bool, "Invalid Serial?"=w614:bool, "Last Test Result"=w609:bool, "Rerun?"=w608:bool)
          n337 = case "New Serial?" shown="False" w615 {
            tunnel: w618 -> [w624 w640]
            tunnel: [w623 w640] -> w617
            tunnel: w616 -> [w622 w643]
            tunnel: w614 -> [w621 _]
            tunnel: [w620 w639] -> w613
            tunnel: w612 -> [w619 w639]
            tunnel: w611 -> [w625 w642]
            tunnel: [w625 w641] -> w610
            tunnel: w609 -> [_ w638]
            tunnel: w608 -> [_ w637]
            tunnel: w607 -> [w626 w636]
            tunnel: [w626 w635] -> w606
            frame True {
              n338 = case "Invalid Serial?" shown="False" w621 {
                tunnel: w624 -> [w630 w631]
                tunnel: [w629 w631] -> w623
                tunnel: w622 -> [w628 w634]
                tunnel: [w627 w633] -> w620
                tunnel: w619 -> [w627 w632]
                frame False {
                  n339 = Build Array (concatenate)(w630, w628) -> (w629:T5[])
                }
                frame True {
                  n340 = Build Array (concatenate)(w632, w634) -> (w633:T5[])
                }
              }
            }
            frame False {
              n341 = case "Last Test Result?" shown="False" w638 {
                tunnel: w636 -> [w647 w653]
                tunnel: [w646 w653] -> w635
                tunnel: w643 -> [w645 w656]
                tunnel: [w648 w655] -> w641
                tunnel: w642 -> [w648 w654]
                tunnel: w637 -> [w644 _]
                frame False {
                  n342 = case "Rerun?" shown="True" w644 {
                    tunnel: w647 -> [w649 w652]
                    tunnel: [w649 w651] -> w646
                    tunnel: w645 -> [_ w650]
                    frame False {
                    }
                    frame True {
                      n343 = Build Array (concatenate)(w652, w650) -> (w651:T5[])
                    }
                  }
                }
                frame True {
                  n344 = Build Array (concatenate)(w654, w656) -> (w655:T5[])
                }
              }
            }
          }
        }
      }
      frame Disabled {
        w657 = T5[] []
        # "Station 4"
        # "Station 3"
        # "Station 2"
        # "Station 1"
        n345 = for {
          tunnel: w662 -> [w673] mode=indexing
          shift-right: [w674] -> w661
          shift-left: w657 -> [w675]
          shift-right: [w670] -> w660
          shift-left: w657 -> [w669]
          shift-right: [w663] -> w659
          shift-left: w657 -> [w664]
          shift-right: [w667] -> w658
          shift-left: w657 -> [w668]
          n346 = Unbundle By Name(w673) -> ("Robot Task"=w672:T6, "Invalid Serial?"=w671:bool, "Last Test Result"=w666:bool, "Rerun?"=w665:bool)
          n347 = case "New Serial?" shown="\"Unload\", Default" w672 {
            tunnel: w675 -> [w679]
            tunnel: [w678] -> w674
            tunnel: w673 -> [w677]
            tunnel: w671 -> [_]
            tunnel: [w676] -> w670
            tunnel: w669 -> [w676]
            tunnel: w668 -> [w680]
            tunnel: [w680] -> w667
            tunnel: w666 -> [_]
            tunnel: w665 -> [_]
            tunnel: w664 -> [w681]
            tunnel: [w681] -> w663
            frame "Unload", Default {
              n348 = Build Array (concatenate)(w679, w677) -> (w678:T5[])
            }
          }
        }
      }
    }
    "Load Serial Tasks" <- w597
    "Invalid Serial Tasks" <- w596
    "Rerun Serial Tasks" <- w595
    "Unload Serial Tasks" <- w594
    n349 = call "ALTS-2015 Task at Station.vi"("Options"=ALTS-2015_Task_at_Station_Options."Read All") -> ("Tasks @ All Stations"=w576:T5[])  [unwired: 8 in, 2 out]
    n350 = Index Array(array=w576) -> (element #1=→"Current Station 1 Task":T5, element #2=→"Current Station 2 Task":T5, element #3=→"Current Station 3 Task":T5, element #4=→"Current Station 4 Task":T5)  [unwired: 4 in]
    n351 = Array Size(array=w597) -> (size(s)=w588:i32)
    "# Load Serial Tasks" <- w588
    n352 = Array Size(array=w596) -> (size(s)=w589:i32)
    "# Invalid Serial Tasks" <- w589
    n353 = Array Size(array=w595) -> (size(s)=w590:i32)
    "# Rerun Serial Tasks" <- w590
    n354 = Array Size(array=w594) -> (size(s)=w591:i32)
    "# Unload Serial Tasks" <- w591
    n355 = global read "ALTS-2015 Global Variables.vi" "Exit Troubleshooter VI"() -> (w593:bool)
    n356 = Not Equal To 0?(x=w588) -> (x != 0?=w587:bool)
    n357 = Not Equal To 0?(x=w589) -> (x != 0?=w584:bool)
    n358 = Not Equal To 0?(x=w590) -> (x != 0?=w585:bool)
    n359 = Not Equal To 0?(x=w591) -> (x != 0?=w586:bool)
    n360 = Select(t=w583, s=w587, f=w582) -> (s? t:f=w580:u32)
    n361 = Select(t=w583, s=w584, f=w582) -> (s? t:f=w579:u32)
    n362 = Select(t=w583, s=w585, f=w582) -> (s? t:f=w581:u32)
    n363 = Select(t=w583, s=w586, f=w582) -> (s? t:f=w578:u32)
    n364 = property on="# Load Serial Tasks" class="DigNum (strict)"("Label.BG Color"=w580, "Label.FG Color"=w580) -> ()  [unwired: 2 in, 2 out]
    n365 = property on="# Rerun Serial Tasks" class="DigNum (strict)"("Label.BG Color"=w581, "Label.FG Color"=w581) -> ()  [unwired: 2 in, 2 out]
    n366 = property on="# Unload Serial Tasks" class="DigNum (strict)"("Label.BG Color"=w578, "Label.FG Color"=w578) -> ()  [unwired: 2 in, 2 out]
    n367 = property on="# Invalid Serial Tasks" class="DigNum (strict)"("Label.BG Color"=w579, "Label.FG Color"=w579) -> ()  [unwired: 2 in, 2 out]
  }
